vi "MainPannelFastEnabled - Copy.vi"() -> ()   [LabVIEW 2020]
uses:
  Digi/Controls/DigiMachineStates.ctl
  Digi/Digitizer_StatesMain.ctl
  <vilib>/userdefined/High Color/nirio_resource_hc.ctl
  Stage/New/StageOptions.ctl
  FileStore/Data Save State.ctl
  Gen/Generator_States.ctl
  <vilib>/Heliosphere Research LLC/Advanced Plotting Toolkit/properties/Colormap_Map.ctl
  <vilib>/Native 3D Graph/xcontrol/3DPC_SurfacePlot.xctl
  WaveClusterPacket.ctl
  <vilib>/UPVI/lvhdf5/library.llb/HDF5 Ref.ctl
  LongShotStates.ctl
  ImageCluster.ctl
  <vilib>/Platform/TimedLoop/XDataNode/timing_clust.ctl
  <vilib>/Platform/TimedLoop/XDataNode/nitl_modes.ctl
  <vilib>/Platform/TimedLoop/XDataNode/wakeup.ctl
  Stage/New/SettingCtrlOptions.ctl
  Stage/New/PosCtrlOptions.ctl
  Digi/Controls/FPGA VI Reference.ctl
  <extravilib>/ChannelInstances/Tag-bool/Read With Abort.vi
  <extravilib>/ChannelInstances/Tag-bool/Write.vi
  <extravilib>/ChannelInstances/Tag-bool/Write With Abort.vi
  <extravilib>/ChannelInstances/Tag-bool/Instantiate.vi
  <extravilib>/ChannelInstances/Tag-bool/EndpointRead.vi
  <vilib>/FPGAPlugInAG/PXIe-7962R/niLvFpga_Open_PXIe-7962R.vi
  <vilib>/rvi/interface/common/dynamic/niFpgaDynamicAddResources.vi
  <vilib>/FPGAPlugInAG/Dynamic/niLvFpga_Close_Dynamic.vi
  <extravilib>/ChannelInstances/Tag-bool/Endpoint.vi
  <vilib>/Platform/TimedLoop/XDataNode/XDataNode.xnode
  <vilib>/rvi/interface/nirviOpenFPGA/nirviOpenFPGA.xnode
  FPGA Bitfiles/DigitizerFPGACode(Fully_Functional)_v3.lvbitx
  <vilib>/rvi/interface/nirviCloseFPGA/nirviCloseFPGA.xnode
  <instrlib>/_niInstr/Basic Elements/v1/FPGA/niInstr Basic Elements v1 FPGA.lvlib
  <vilib>/Platform/TimedLoop/XDataNode/XDNodeRunTimeDep.lvlib
  Stage/libximc.lvlib
  <extravilib>/ChannelInstances/Tag-bool.lvlib
  <vilib>/Heliosphere Research LLC/Advanced Plotting Toolkit/Advanced Plotting Toolkit.lvlib
panel:
  in  "Save Img":bool
  out "Image Display":dbl[][](graph)
  in  "Colormap Selector":T1(ring)=enum."gray"
  in  "LongShot":bool
  out "Z Open?":bool
  out "Z Position":dbl format="%#.3g"
  in  "Z_Stop":bool
  in  "Z_MoveDown":bool
  in  "Z_Move Up":bool
  in  "Z_Step":dbl
  in  "Reset Button":bool
  in  "LogMode":bool
  in  "Start Digitizer UI Bttn":bool
  out "Max Index (s)":dbl format="%#_3p"
  out "Max Val (V)":dbl format="%#_3p"
  in  "Delay_Scroll_Range":dbl=2.0 caption="Range"
  in  "FineDelayControl":dbl(slide)=1.0 step=0.1 scale=-2.0..2.0
  in  "Amplitude Range":cluster{"Slider 1":dbl, "Slider 1":dbl}(slide)={"Slider 1"=1.0, "Slider 1"=1.6299559471365639} scale=-2.5..2.5
  in  "Pause Triggger":bool caption="Pause"
  in  "Delay(us)":sgl min=0 step=0.1 format="%#_4g"
  in  "Time Division":u8(slide)=1 max=2 step=1 scale=0.0..2.0
  in  "Amplitude \nAveraging":u16(slide)=1 caption="Amplitude Averaging" scale=0.0..7.0 scale format="%#.2g"
  in  "Record Size":u16=1024
  in  "RIO Resource":T2="PXI1Slot2"
  out "Configured?":bool
  out "TIS Configured?":bool
  out "Range (Vpp)":dbl=1.3
  out "Digitizer On":bool
  out "Waveform [LIVE]":cluster{"Start Time":dbl, dbl, ext[]}(graph)
  in  "TriggerDigi":bool
  in  "Scanning":bool
  in  "Single Shot":bool
  in  "LIVE":bool
  in  "Transducer Freq (Hz)":u64
  in  "Temperature (C)":dbl
  in  "Remarks":string
  in  "Immersion Medium":string
  in  "EXIT APP":bool
  in  "Save to File":bool=TRUE caption="Checkbox"
  out "No Trig Miss":bool
  in  "FileName":string
  in  "File Store Directory":path
  out "File Open?":bool
  out "X Step Size (R)":sgl format="%#_2g"
  out "Y Step Size (R)":sgl format="%#_2g"
  out "Scan Time (Approx.)":string
  out "Total Pixels":i32
  out "Moving?":bool
  out "Stage Position":cluster{sgl[], sgl[]}(graph) caption="XY Graph - Dark"
  in  "X Position Abs":dbl caption="X Position"
  in  "Y Position Abs":dbl caption="Y Position"
  out "Line Count":i32=6 caption="Y Pixels"
  out "Pixel Count":i32=6 caption="X Pixels"
  in  "X Start":sgl
  in  "X End":sgl=10.0
  in  "Y Start":sgl
  in  "Y End":sgl=8.0
  in  "Y Step Size":sgl=0.5
  in  "X Step Size":sgl=0.5
  in  "Scan Mode":enum16{"Raster", "Serpentine"}(ring)
  in  "Speed Control (mm/s)":sgl(slide)=4.0 min=0.1 scale=0.1..5.0
  in  "AbsMove":bool
  in  "Outline":bool
  in  "Start Stage":bool
  in  "Stop Motion":bool
  in  "Zero":bool
  in  "Right":bool
  in  "Left":bool
  in  "Move to Start":bool
  in  "Down":bool
  in  "Up":bool
  out "X Position":dbl format="%#.3g"
  out "Y Position":dbl format="%#.3g"
  in  "Move Step":dbl=1.0
  in  "Stop Stage":bool
  out "Controller Open?":bool
  in  "Developer Options Control":T3(tab)
  in  "Stop Gen App":bool
  out "Gen State":T4
  out "Error Out Gen":errorcluster
  in  "Send vi Trig":bool
  out "Gain":dbl
  out "Offset Factor":dbl
  out "Amplitudes":dbl[](array[numeric]) format="%.2f"
  out "Sampling Frequency (Hz)":u64
  out "Waves per Pixel":u32
  in  "Ext/nViTrig":bool=TRUE
  in  "Machine Mode":T5(ring)=enum."Normal"
  in  "Stop Stage App":bool
  out "Error Out Stage":errorcluster
  in  "Next Coordinate Index":i32
  in  "EdgePt/nPixelMap":bool=TRUE
  out "Coordinate Array":sgl[][](array[numeric])
  out "Step Sizes":sgl[](array[numeric])
  out "Peripheral Coordis":sgl[][](array[numeric])=[[0.0, 0.0], [1.8, 0.0], [3.6, 0.0], [5.3999996, 0.0], [7.2, 0.0], [9.0, 0.0], [9.0, 2.0], [7.2, 2.0], [5.3999996, 2.0], [3.6, 2.0], [1.8, 2.0], [0.0, 2.0], [0.0, 4.0], [1.8, 4.0], [3.6, 4.0], [5.3999996, 4.0], [7.2, 4.0], [9.0, 4.0], [9.0, 6.0], [7.2, 6.0], [5.3999996, 6.0], [3.6, 6.0], [1.8, 6.0], [0.0, 6.0], [0.0, 8.0], [1.8, 8.0], [3.6, 8.0], [5.3999996, 8.0], [7.2, 8.0], [9.0, 8.0], [9.0, 10.0], [7.2, 10.0], [5.3999996, 10.0], [3.6, 10.0], [1.8, 10.0], [0.0, 10.0]]
  in  "Correction Table Path (Hidden)":path
  out "Serial nos":u32[](array[numeric])
  out "Calibration":cluster{dbl, "MicrostepMode":u32}[](array[cluster])
  out "IDs":i32[](array[numeric])
  in  "X Max Stage":dbl=220.0 format="%#_13g"
  in  "Y Maximum":dbl=220.0
  out "Stage Status":T6
  out "Wave Count Zero":bool
  in  "CountReset":bool
  in  "Trigger Digi Single":bool
  in  "Start Digi":bool
  in  "Stop Digi App":bool caption="Stop Digi \nApplication"
  in  "Digi Machine Mode":T7=enum."Single Shot Mode"
  out "Waves Count":u32
  in  "Imaging":bool
  out "Digi State":T8
  out "nDigiLoopRunning":bool
  out "error out Digi":errorcluster
  out "Wave out packet":T9
  out "Error Out FileIO":errorcluster
  in  "Done Recording":bool
  in  "Record Data":bool
  in  "Open File":bool
  in  "Stop File App":bool
  out "FileStore State":T10
  out "Scan Running":bool=TRUE
  out "Scan Complete":bool=TRUE
  out "AmplitudeArray":dbl[](array[numeric])
  out "IndexArray":dbl[](array[numeric])
  in  "Map":T11
  in  "ColorBar":bool
  in  "Axis":bool
  out "Scanned Image":picture
  out "Topography Plot":refnum<class "Base Datatype.lvclass">[](xcontrol)
  in  "LongShotTimes":u8
  out "FilenameSimeStamped":string
  out "FileDirectoryFinal":path
  in  "Generator  Port":refnum<k15>
  out "Actual Sample Rate":dbl format="%#_6p"
  in  "Use Default Wave Settings":bool caption="Checkbox"
  in  "Start Gen":bool
  in  "stop Gen":bool
  out "Generator On":bool
  out "Input Waveform":dbl[](graph)
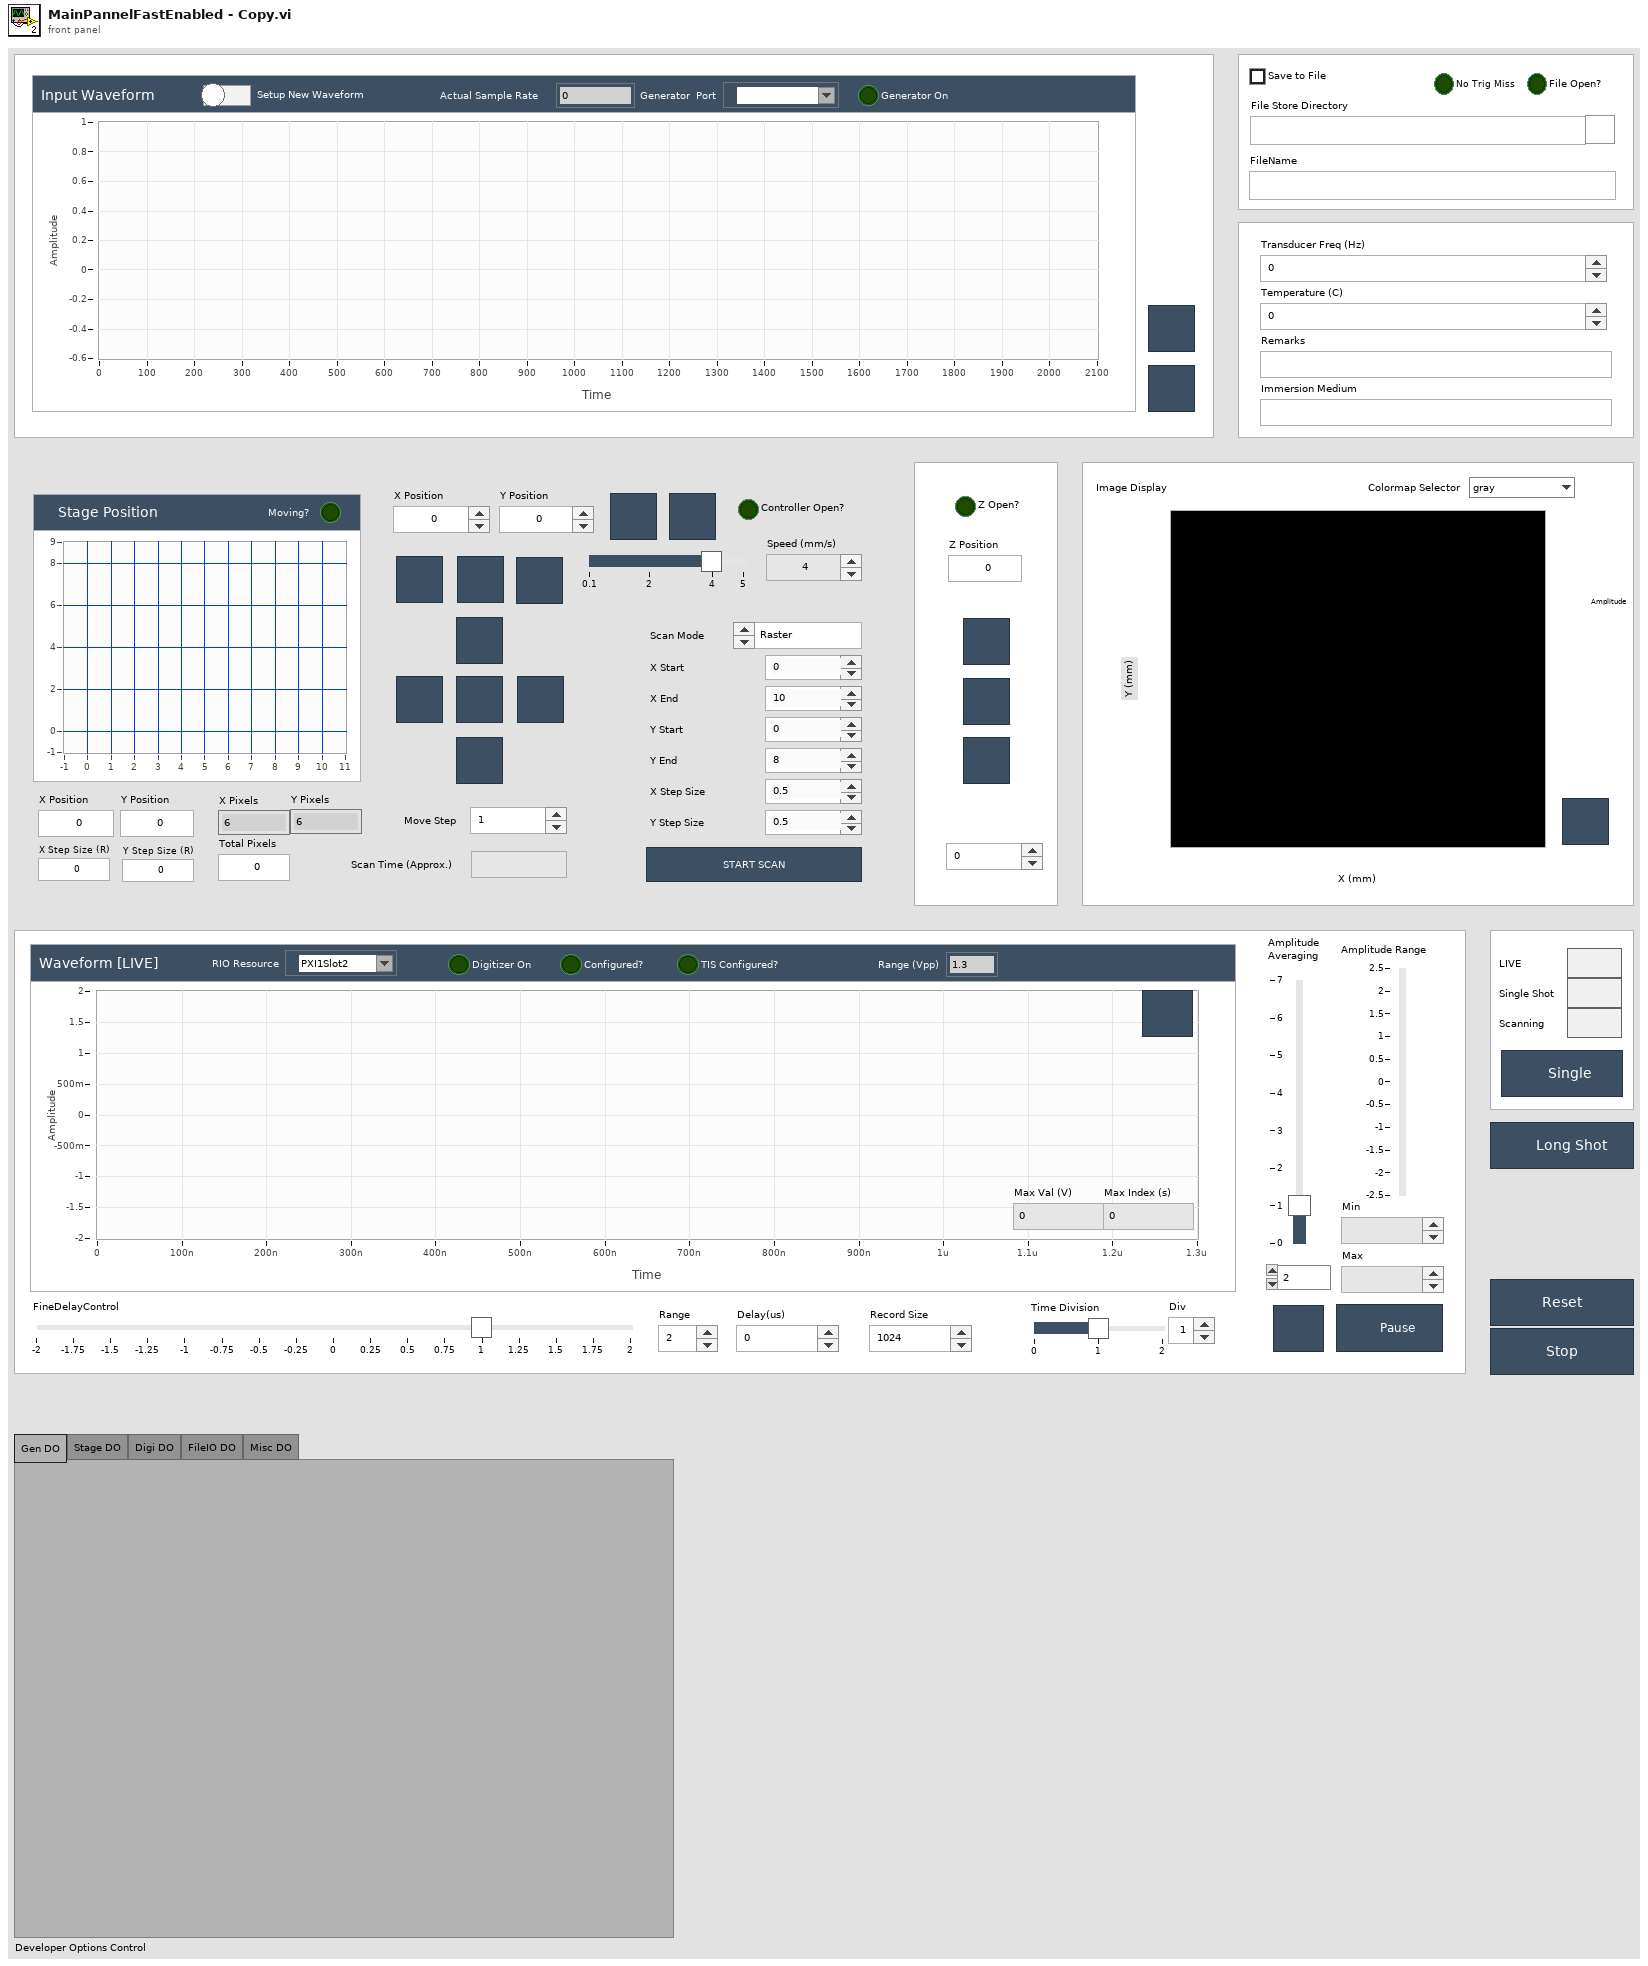
[diagram p1: front panel]
types:
  T1 = enum16{"fire", "rainbow", "gray", "inverse gray", "ice", "original"}
  T2 = typedef "nirio_resource_hc.ctl" = tag
  T3 = enum32{"Gen DO", "Stage DO", "Digi DO", "FileIO DO", "Misc DO"}
  T4 = typedef "Generator_States.ctl" = enum16{"Idle", "GenerateWaveArray", "InitGen", "SendVITrig", "CloseGen", "CloseApp"}
  T5 = enum16{"Scanning Mode", "Perimeter Mode", "Normal"}
  T6 = typedef "StageOptions.ctl" = enum16{"Idle", "Init", "Set Speed", "GenerateMotionPoints", "Scan_Start", "Scan_MoveNext", "Scan_SyncSet", "Scan_Get Pos", "Scan_Complete", "Cmd_MoveAbs", "Cmd_CloseControllers", "Cmd_MoveUp", "Cmd_MoveDown", "Cmd_MoveLeft", "Cmd_MoveRight", "Cmd_MoveStart", "Cmd_MoveZero", "Cmd_GetPos", "Cmd_Stop", "Sync_On", "Sync_Off", "Stop Motion", "CloseApplication"}
  T7 = typedef "DigiMachineStates.ctl" = enum16{"Scanning Mode", "Live Mode", "Single Shot Mode", "Idle Mode"}
  T8 = typedef "Digitizer_StatesMain.ctl" = enum16{"Idle", "Init", "SetParam", "VITrig", "Read", "CloseDigi", "CloseApp"}
  T9 = typedef "WaveClusterPacket.ctl" = cluster{"Wave Count":u32, "Wave":i16[]}
  T10 = typedef "Data Save State.ctl" = enum16{"Idle", "Open File", "Write Attributes", "Append Data", "Close File", "Close App"}
  T11 = typedef "Advanced Plotting Toolkit.lvlib/Colormap_Map.ctl" = enum16{"Automatic", "Rainbow", "Hot and Cold", "White-Black", "White-Blue", "White-Green", "White-Red", "Fire", "Water", "Earth", "Air", "Pastel", "Banded", "Stepped"}
  T12 = typedef "ImageCluster.ctl" = cluster{"Wave Count":i16, "Amplitude":i32, "Index":i32}
  T13 = typedef "LongShotStates.ctl" = enum16{"Idle", "Start Gen", "Set Digi Mode", "Clear Wave Count", "Set Initial Param", "Set Param", "Take Shot", "UpdateParam", "Show Data"}
  T14 = typedef "HDF5 Ref.ctl" = refnum<k1>
  T15 = typedef "XDNodeRunTimeDep.lvlib/timing_clust.ctl" = cluster{"Expected End [f-1]":u64, "Actual End [f-1]":u64, "Finished Late? [f-1]":bool, "Expected End [i-1]":u64, "Actual End [i-1]":u64, "Finished Late? [i-1]":bool, "Expected Start [i]":u64, "Actual Start [i]":u64, "Expected Start [f]":u64, "Actual Start [f]":u64, "Source Name":string, "Structure Name":string, "Period":i64, "Deadline":i64, "Offset":i64, "Start":i64, "Priority":i32, "Timeout":i32, "Mode":T16, "Wakeup Reason":T17, "Error":errorcluster, "Source Type":string, "Secondary Source Type":string, "Global End Time":u64, "Global Start Time":u64, "Frame Duration":u64, "Iteration Duration":u64, "Assigned CPU":i32, "I/O Scan Engine Mode":u32}
  T16 = typedef "XDNodeRunTimeDep.lvlib/nitl_modes.ctl" = enum32{"No Change", "Process missed periods, maintain original phase", "Discard missed periods, maintain original phase", "Process missed periods, ignore original phase", "Discard missed periods, ignore original phase"}
  T17 = typedef "XDNodeRunTimeDep.lvlib/wakeup.ctl" = enum32{"Normal", "Aborted", "Asynchronous wakeup", "Timing source error", "Timed loop error", "Timeout"}
  T18 = typedef "SettingCtrlOptions.ctl" = enum16{"Set X", "Set Y", "Set X and Y", "Get Settings", "None"}
  T19 = typedef "PosCtrlOptions.ctl" = enum16{"Move X", "Move Y", "Both X and Y", "Read Pos", "None"}
  T20 = typedef "imagedata.ctl" = cluster{"image type":i32, "image depth":i32, "image":u8[], "mask":u8[], "colors":u32[], "Rectangle":cluster{"left":i16, "top":i16, "right":i16, "bottom":i16}}
  T21 = typedef "FPGA VI Reference.ctl" = refnum<k20>
  T22 = typedef "Tag-bool.lvlib/))Channel.ctl" = refnum<queue>
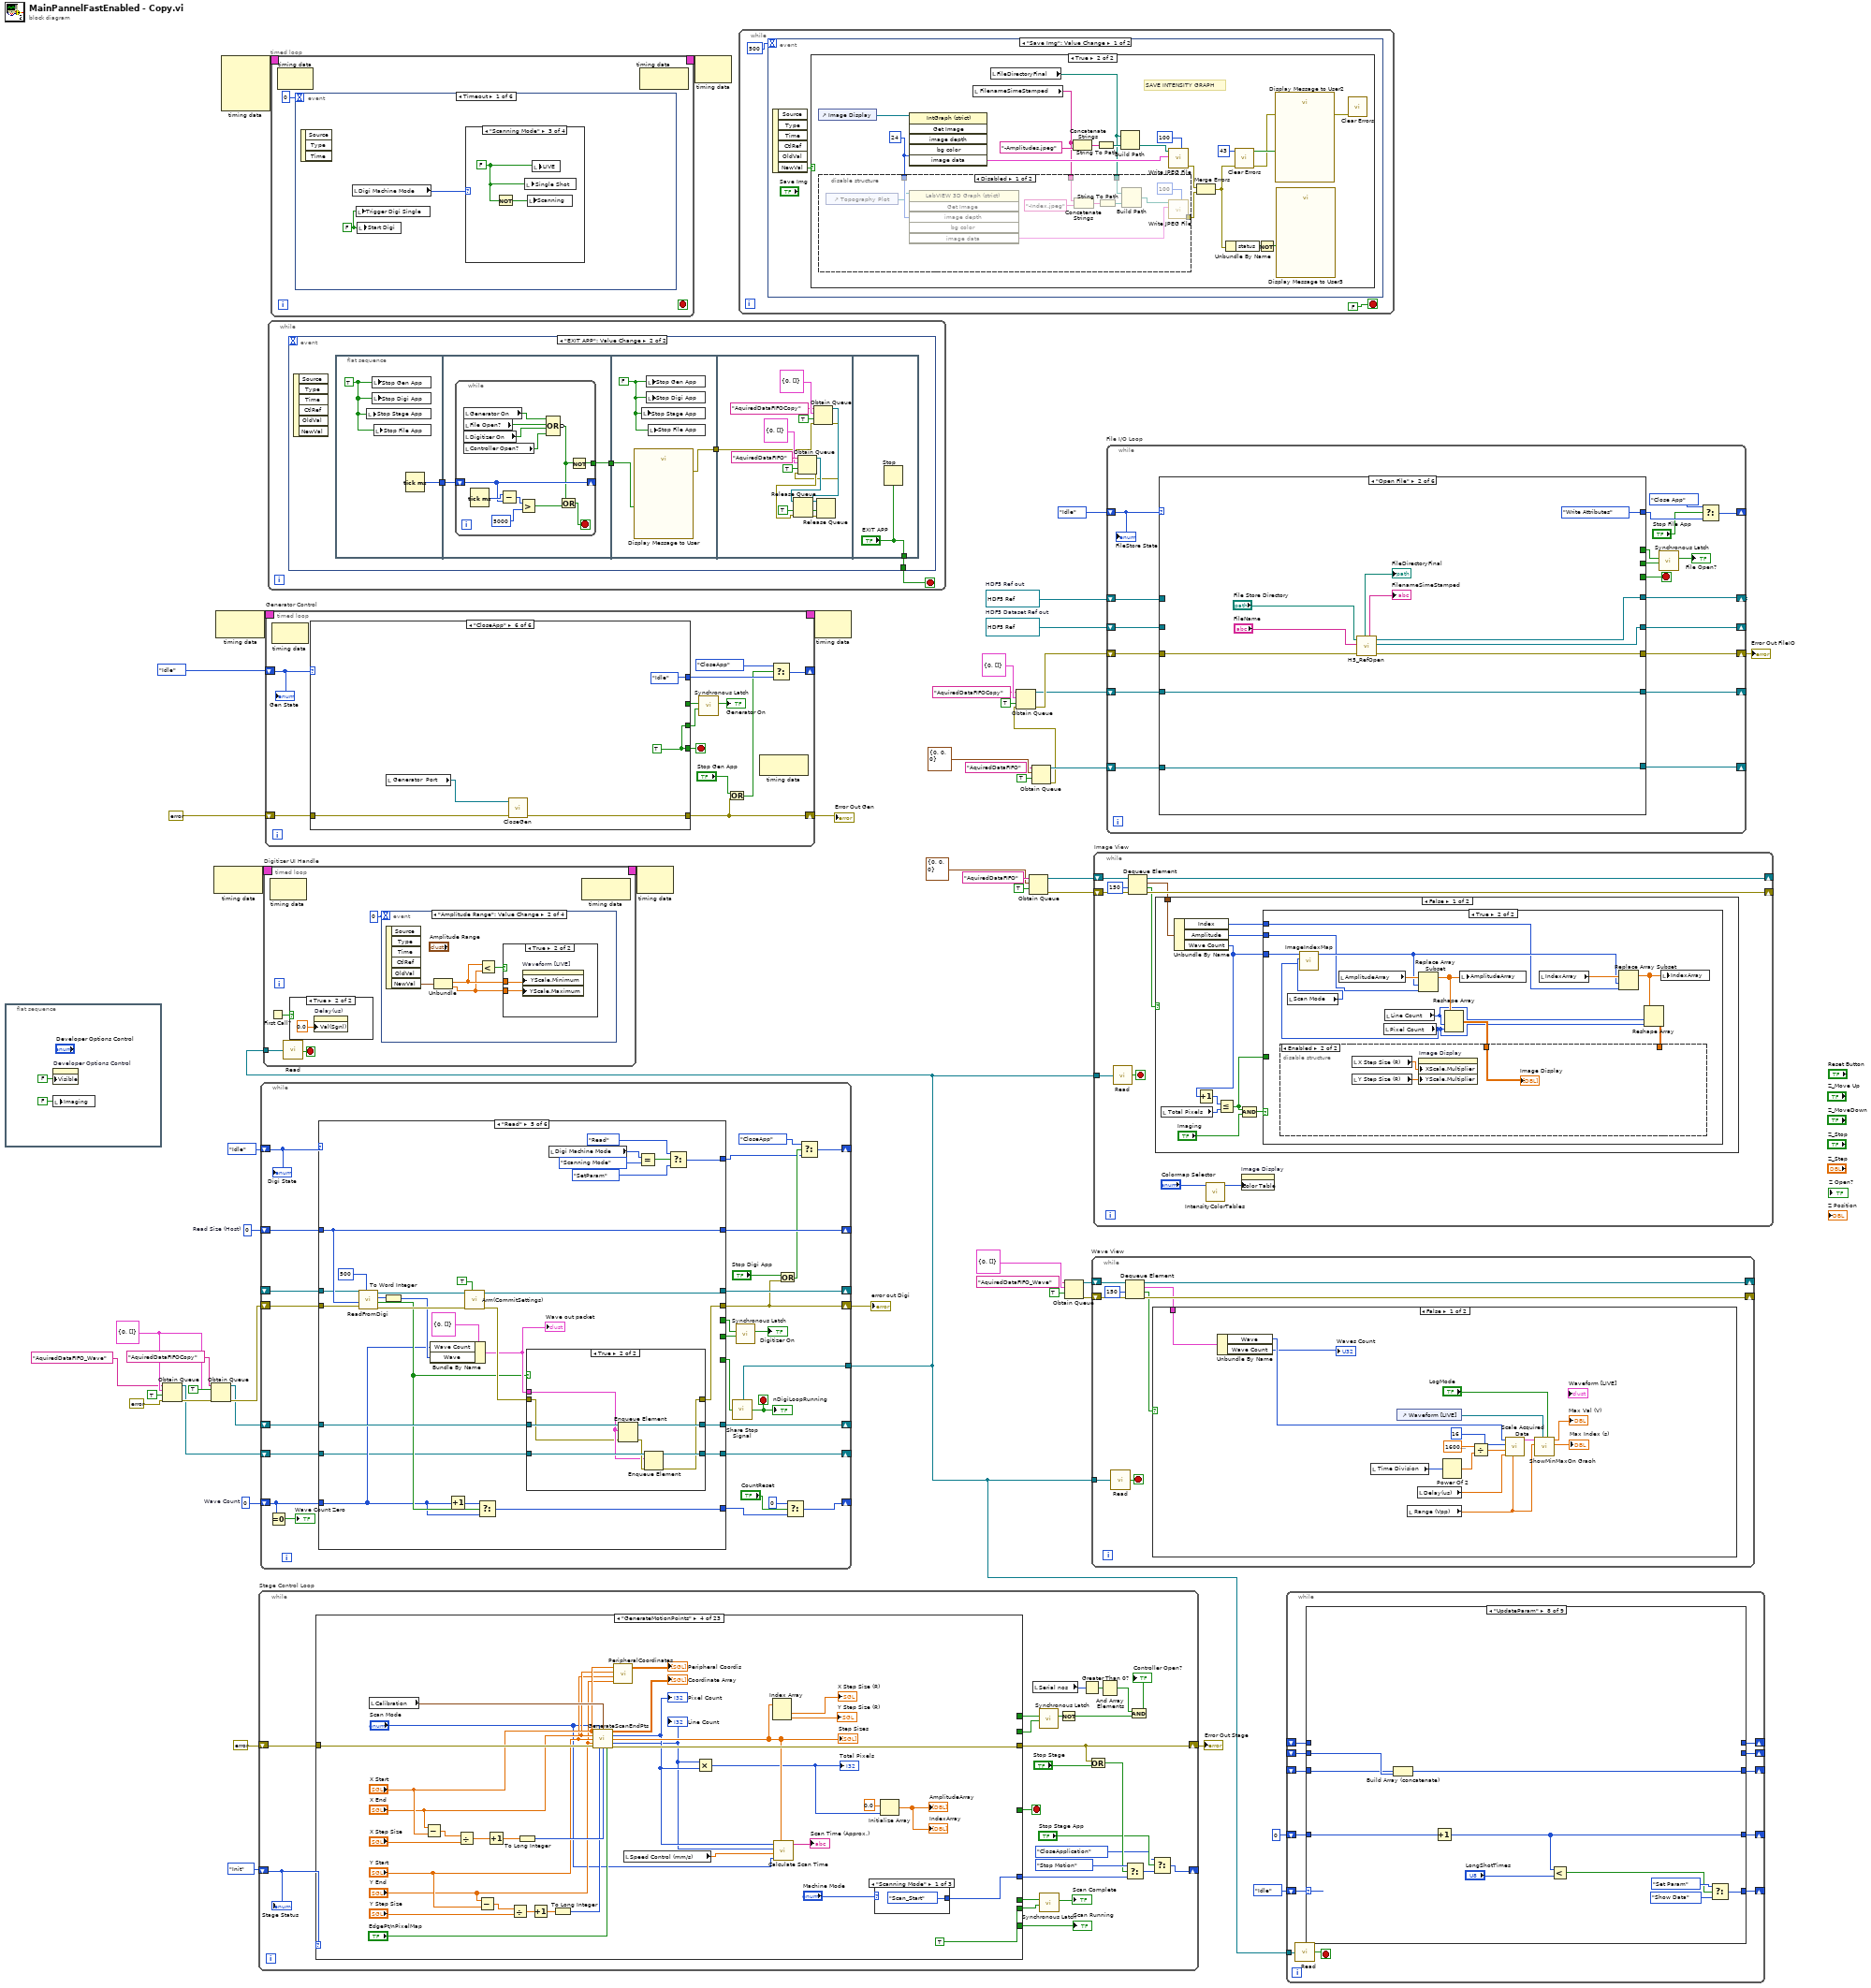
[diagram p0: block diagram]
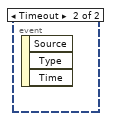
[diagram p4: hidden frame]
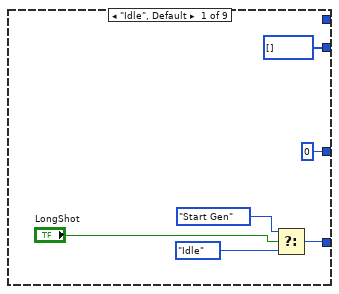
[diagram p5: hidden frame]
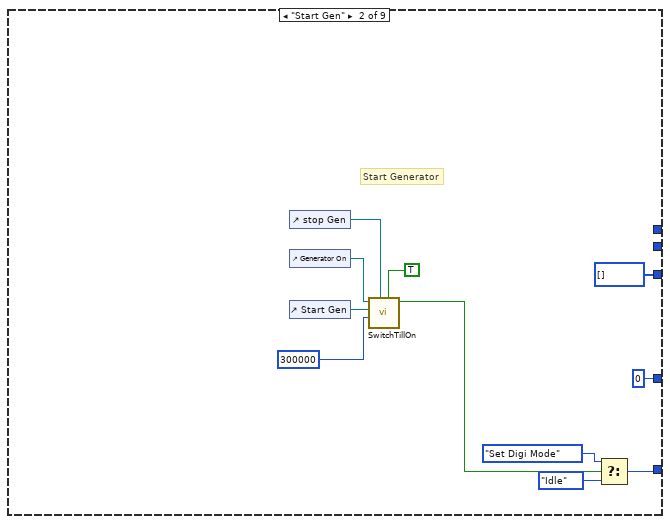
[diagram p6: hidden frame]
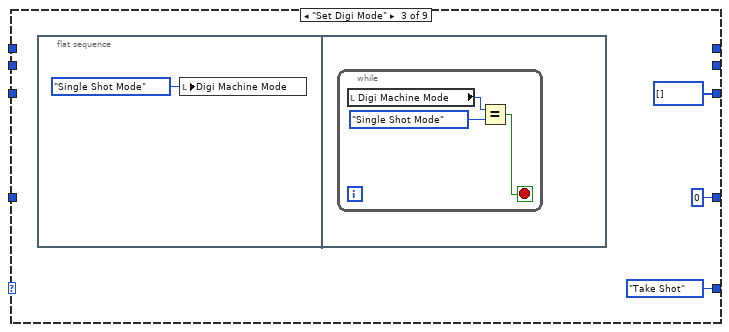
[diagram p7: hidden frame]
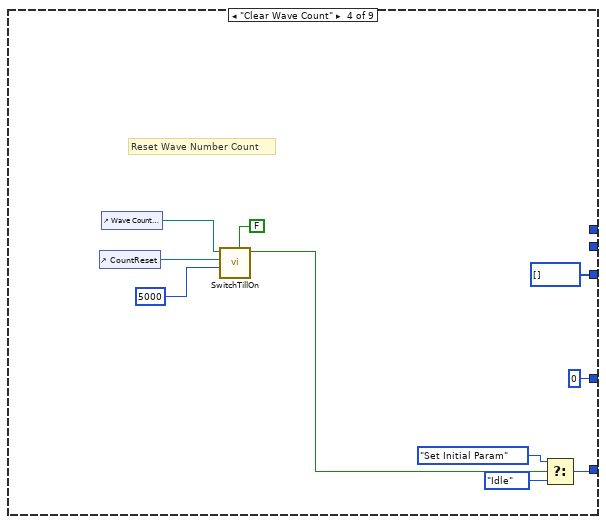
[diagram p8: hidden frame]
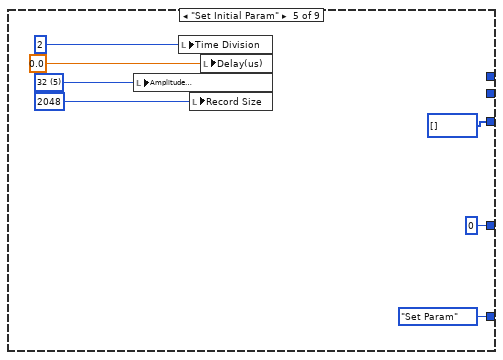
[diagram p9: hidden frame]
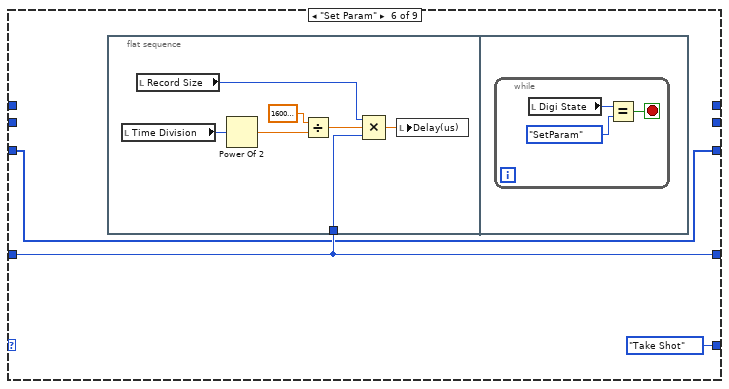
[diagram p10: hidden frame]
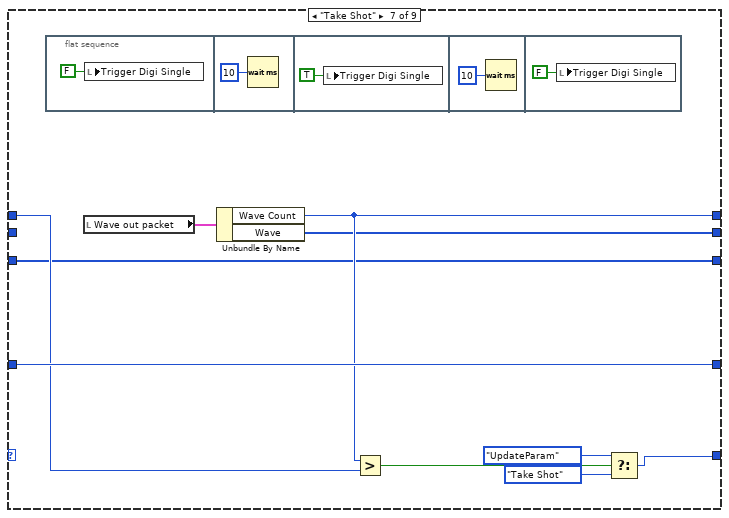
[diagram p11: hidden frame]
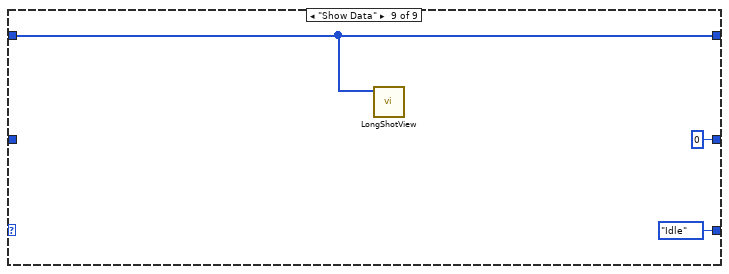
[diagram p12: hidden frame]
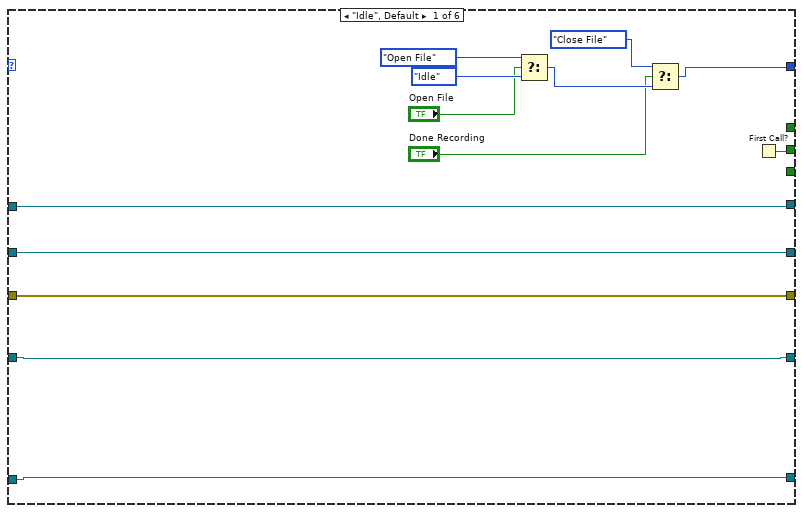
[diagram p14: hidden frame]
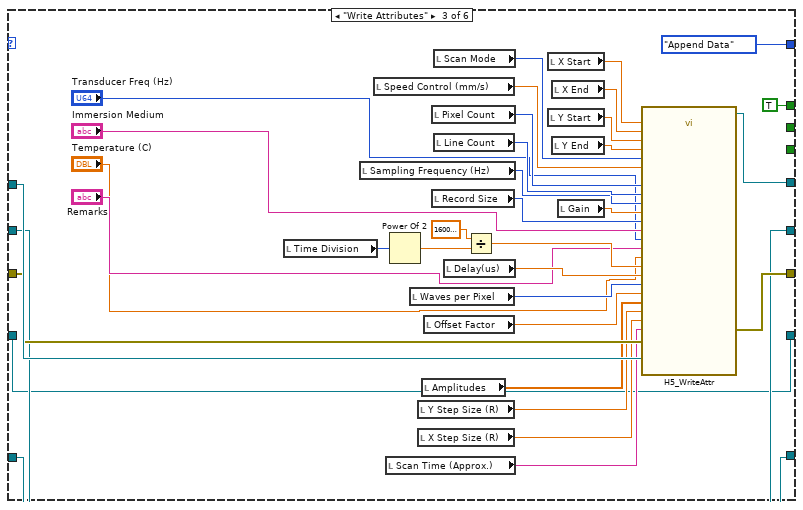
[diagram p15: hidden frame]
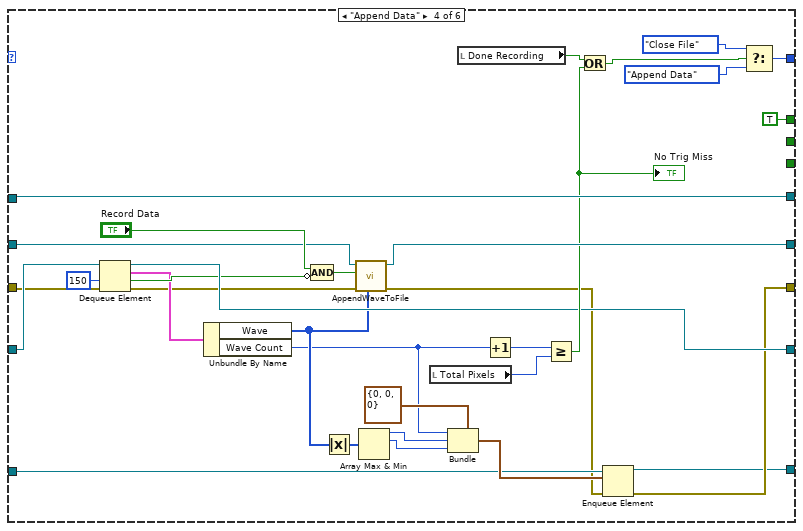
[diagram p16: hidden frame]
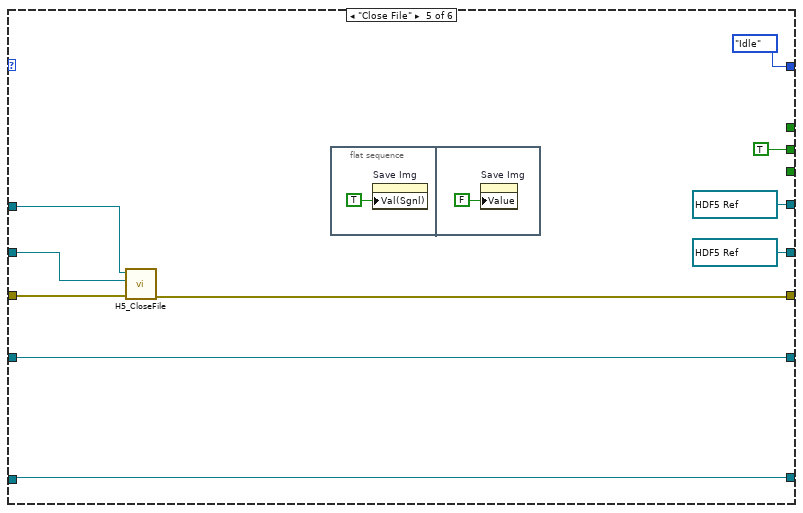
[diagram p17: hidden frame]
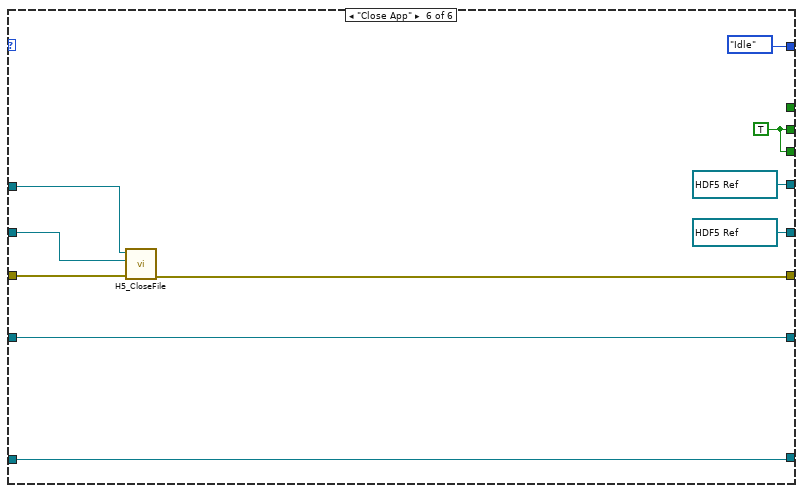
[diagram p18: hidden frame]
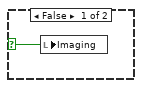
[diagram p19: hidden frame]
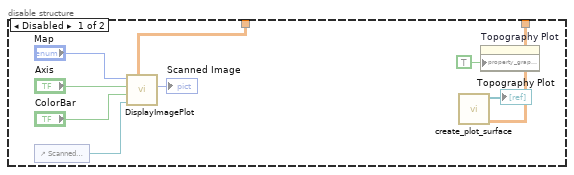
[diagram p20: hidden frame]
diagram:
  w31 = u16 0  # Wave Count
  w18 = T9 {"Wave Count"=0, "Wave"=[]} ("input cluster")
  w37 = T14 refnum items=["HDF5 Ref"]  # HDF5 Dataset Ref out
  w38 = T14 refnum items=["HDF5 Ref"]  # HDF5 Ref out
  w48 = u16 0  # Read Size (Host)
  n1 = flat-sequence {
    frame #0 {
      n2 = property on="Developer Options Control" class="TabCtl (strict)"("Visible"=FALSE) -> ()  [unwired: 2 in, 2 out]
      n3 = local write "Imaging"(FALSE ("Imaging")) -> ()
    }
  }
  n4 = Obtain Queue(name (unnamed)="AquiredDataFIFO_Wave", element data type=w18, create if not found? (T)=TRUE, error in (no error)=errorcluster {"status"=FALSE, "code"=0, "source"=""}) -> (queue out=w19:refnum<queue>, error out=w22:errorcluster)  [unwired: 1 in, 1 out]
  n5 = Obtain Queue(name (unnamed)="AquiredDataFIFOCopy", element data type=w18, create if not found? (T)=TRUE, error in (no error)=w22) -> (queue out=w33:refnum<queue>, error out=w34:errorcluster)  [unwired: 1 in, 1 out]
  n6 = node-c288() -> (w51:T15)  [unwired: 1 in]
  n7 = node-c288() -> (w45:T15)  [unwired: 1 in]
  n8 = node-c288() -> (w24:T15)  [unwired: 4 in]
  n9 = while "Stage Control Loop" {
    shift-right: [w68] -> _
    shift-left: StageOptions."Init" -> [w79]
    shift-right: [w76] -> w11
    shift-left: errorcluster {"status"=FALSE, "code"=0, "source"=""} ("error out") -> [w77]
    stop <- w69 stop-if-true
    n10 = case shown="\"GenerateMotionPoints\"" w79 {
      tunnel: [w84 w180 w203 w240 w245 w375 w390 w404 w444 w466 w475 w482 w493 w503 w513 w522 w530 w545 w551 w562 w571 w579 w590] -> w76
      tunnel: w77 -> [w84 w178 w204 w239 w247 w376 w391 w405 w442 w467 w476 w481 w494 w504 w514 w523 w531 w546 w550 w563 w572 w578 w589]
      tunnel: [w83 StageOptions."Set Speed" StageOptions."GenerateMotionPoints" w224 w248 w366 StageOptions."Scan_MoveNext" w401 StageOptions."Idle" StageOptions."Idle" StageOptions."Idle" StageOptions."Idle" StageOptions."Idle" StageOptions."Idle" StageOptions."Idle" StageOptions."Idle" StageOptions."Idle" StageOptions."Idle" StageOptions."Idle" StageOptions."Idle" StageOptions."Idle" StageOptions."Idle" StageOptions."Idle"] -> w74
      tunnel: [_ _ _ _ _ _ _ _ _ _ _ _ _ _ _ _ _ _ _ _ _ w575 w585] -> w72
      tunnel: [_ w181 _ _ _ _ _ _ _ _ _ _ _ _ _ _ _ _ _ _ _ _ _] -> w70
      tunnel: [_ _ _ _ _ _ _ _ _ _ _ _ _ _ _ _ _ _ _ _ _ _ w585] -> w69
      tunnel: [_ _ _ _ _ _ _ _ TRUE ("X SyncOut Enabled") _ _ _ _ _ _ _ _ _ _ _ _ _ _] -> w59
      tunnel: [TRUE ("EdgePt/nPixelMap") TRUE ("EdgePt/nPixelMap") TRUE ("EdgePt/nPixelMap") TRUE ("EdgePt/nPixelMap") TRUE ("EdgePt/nPixelMap") _ _ _ _ _ _ _ _ _ _ _ _ _ _ _ _ _ _] -> w57
      tunnel: [_ _ _ _ _ TRUE ("Moving?") TRUE ("Moving?") w392 FALSE ("Moving?") _ _ _ _ _ _ _ _ _ _ _ _ _ _] -> w56
      frame "Idle", Default {
        n11 = First Call?() -> (First Call?: T/F=w81:bool)
        n12 = event shown="[1] \"Up\": Value Change" {
          selector: _ -> [_ _ _ _ _ _ _ _ _ _ _ _ _]
          dyn-events: _ -> [_ _ _ _ _ _ _ _ _ _ _ _ _]
          timeout: 100 -> [_ _ _ _ _ _ _ _ _ _ _ _ _]
          tunnel: [w87 StageOptions."Cmd_MoveUp" StageOptions."Cmd_MoveDown" StageOptions."Cmd_MoveStart" StageOptions."Cmd_MoveLeft" StageOptions."Cmd_MoveRight" StageOptions."Cmd_MoveZero" StageOptions."Cmd_Stop" StageOptions."GenerateMotionPoints" StageOptions."GenerateMotionPoints" StageOptions."Set Speed" w159 StageOptions."Cmd_MoveAbs"] -> w83
          event Timeout {
            n13 = event-data() -> ()  [unwired: 1 in, 3 out]
            n14 = local read "Controller Open?"() -> (w88:bool)
            n15 = case shown="False" w88 {
              tunnel: [StageOptions."Init" StageOptions."Cmd_GetPos"] -> w87
              frame False {
              }
              frame True {
              }
            }
          }
          event "Up": Value Change {
            w91 = 0.0  # Y Start
            w93 = sgl 0.0  # X Start
            w96 = 1.0  # Offset
            n16 = event-data() -> ()  [unwired: 1 in, 6 out]
            n17 = local read "X Max Stage"() -> (w94:dbl)
            n18 = local read "Y Maximum"() -> (w92:dbl)
            n19 = Add(x=w96, y=w94) -> (x+y=w98:dbl)
            n20 = Subtract(x=w93, y=w96) -> (x-y=w99:dbl)
            n21 = Subtract(x=w91, y=w96) -> (x-y=w95:dbl)
            n22 = Add(x=w92, y=w96) -> (x+y=w97:dbl)
            n23 = Build Array(w93, w94) -> (w101:dbl[])
            n24 = Build Array(w91, w92) -> (w100:dbl[])
            n25 = property on="Stage Position" class="XYGraph (strict)"("XScale.Maximum"=w98, "XScale.Minimum"=w99, "YScale.Maximum"=w97, "YScale.Minimum"=w95, "XScale.MarkerVals[]"=w101, "YScale.MarkerVals[]"=w100) -> ()  [unwired: 2 in, 2 out]
          }
          event "Down": Value Change {
            w103 = 0.0  # Y Start
            w105 = sgl 0.0  # X Start
            w108 = 1.0  # Offset
            n26 = event-data() -> ()  [unwired: 1 in, 6 out]
            n27 = local read "X Max Stage"() -> (w106:dbl)
            n28 = local read "Y Maximum"() -> (w104:dbl)
            n29 = Add(x=w108, y=w106) -> (x+y=w110:dbl)
            n30 = Subtract(x=w105, y=w108) -> (x-y=w111:dbl)
            n31 = Subtract(x=w103, y=w108) -> (x-y=w107:dbl)
            n32 = Add(x=w104, y=w108) -> (x+y=w109:dbl)
            n33 = Build Array(w105, w106) -> (w113:dbl[])
            n34 = Build Array(w103, w104) -> (w112:dbl[])
            n35 = property on="Stage Position" class="XYGraph (strict)"("XScale.Maximum"=w110, "XScale.Minimum"=w111, "YScale.Maximum"=w109, "YScale.Minimum"=w107, "XScale.MarkerVals[]"=w113, "YScale.MarkerVals[]"=w112) -> ()  [unwired: 2 in, 2 out]
          }
          event "Move to Start": Value Change {
            n36 = event-data() -> ()  [unwired: 1 in, 6 out]
          }
          event "Left": Value Change {
            w116 = 0.0  # Y Start
            w118 = sgl 0.0  # X Start
            w121 = 1.0  # Offset
            n37 = event-data() -> ()  [unwired: 1 in, 6 out]
            n38 = local read "X Max Stage"() -> (w119:dbl)
            n39 = local read "Y Maximum"() -> (w117:dbl)
            n40 = Add(x=w121, y=w119) -> (x+y=w123:dbl)
            n41 = Subtract(x=w118, y=w121) -> (x-y=w124:dbl)
            n42 = Subtract(x=w116, y=w121) -> (x-y=w120:dbl)
            n43 = Add(x=w117, y=w121) -> (x+y=w122:dbl)
            n44 = Build Array(w118, w119) -> (w126:dbl[])
            n45 = Build Array(w116, w117) -> (w125:dbl[])
            n46 = property on="Stage Position" class="XYGraph (strict)"("XScale.Maximum"=w123, "XScale.Minimum"=w124, "YScale.Maximum"=w122, "YScale.Minimum"=w120, "XScale.MarkerVals[]"=w126, "YScale.MarkerVals[]"=w125) -> ()  [unwired: 2 in, 2 out]
          }
          event "Right": Value Change {
            w128 = 0.0  # Y Start
            w130 = sgl 0.0  # X Start
            w133 = 1.0  # Offset
            n47 = event-data() -> ()  [unwired: 1 in, 6 out]
            n48 = local read "X Max Stage"() -> (w131:dbl)
            n49 = local read "Y Maximum"() -> (w129:dbl)
            n50 = Add(x=w133, y=w131) -> (x+y=w135:dbl)
            n51 = Subtract(x=w130, y=w133) -> (x-y=w136:dbl)
            n52 = Subtract(x=w128, y=w133) -> (x-y=w132:dbl)
            n53 = Add(x=w129, y=w133) -> (x+y=w134:dbl)
            n54 = Build Array(w130, w131) -> (w138:dbl[])
            n55 = Build Array(w128, w129) -> (w137:dbl[])
            n56 = property on="Stage Position" class="XYGraph (strict)"("XScale.Maximum"=w135, "XScale.Minimum"=w136, "YScale.Maximum"=w134, "YScale.Minimum"=w132, "XScale.MarkerVals[]"=w138, "YScale.MarkerVals[]"=w137) -> ()  [unwired: 2 in, 2 out]
          }
          event "Zero": Value Change {
            w140 = 0.0  # Y Start
            w142 = sgl 0.0  # X Start
            w145 = 1.0  # Offset
            n57 = event-data() -> ()  [unwired: 1 in, 6 out]
            n58 = local read "X Max Stage"() -> (w143:dbl)
            n59 = local read "Y Maximum"() -> (w141:dbl)
            n60 = Add(x=w145, y=w143) -> (x+y=w147:dbl)
            n61 = Subtract(x=w142, y=w145) -> (x-y=w148:dbl)
            n62 = Subtract(x=w140, y=w145) -> (x-y=w144:dbl)
            n63 = Add(x=w141, y=w145) -> (x+y=w146:dbl)
            n64 = Build Array(w142, w143) -> (w150:dbl[])
            n65 = Build Array(w140, w141) -> (w149:dbl[])
            n66 = property on="Stage Position" class="XYGraph (strict)"("XScale.Maximum"=w147, "XScale.Minimum"=w148, "YScale.Maximum"=w146, "YScale.Minimum"=w144, "XScale.MarkerVals[]"=w150, "YScale.MarkerVals[]"=w149) -> ()  [unwired: 2 in, 2 out]
          }
          event "Stop Motion": Value Change {
            n67 = event-data() -> ()  [unwired: 1 in, 6 out]
          }
          event "Start Stage": Value Change {
            n68 = event-data() -> ()  [unwired: 1 in, 6 out]
            n69 = local write "Machine Mode"(T5."Scanning Mode" ("Machine Mode")) -> ()
          }
          event "X Start", "X End", "Y Start", "Y End", "Y Step Size", "X Step Size", "Scan Mode": Value Change {
            n70 = event-data() -> ()  [unwired: 1 in, 6 out]
            n71 = local write "Machine Mode"(T5."Normal" ("Machine Mode")) -> ()
          }
          event "Speed Control (mm/s)": Value Change {
            n72 = event-data() -> ()  [unwired: 1 in, 6 out]
          }
          event "Outline": Value Change {
            n73 = event-data() -> ()  [unwired: 1 in, 6 out]
            n74 = case shown="True" "Outline" {
              tunnel: [StageOptions."Idle" StageOptions."GenerateMotionPoints"] -> w159
              frame False {
              }
              frame True {
                n75 = local write "Machine Mode"(T5."Perimeter Mode" ("Machine Mode")) -> ()
              }
            }
          }
          event "AbsMove": Value Change {
            w163 = 0.0  # Y Start
            w165 = sgl 0.0  # X Start
            w168 = 1.0  # Offset
            n76 = event-data() -> ()  [unwired: 1 in, 6 out]
            n77 = local read "X Max Stage"() -> (w166:dbl)
            n78 = local read "Y Maximum"() -> (w164:dbl)
            n79 = Add(x=w168, y=w166) -> (x+y=w170:dbl)
            n80 = Subtract(x=w165, y=w168) -> (x-y=w171:dbl)
            n81 = Subtract(x=w163, y=w168) -> (x-y=w167:dbl)
            n82 = Add(x=w164, y=w168) -> (x+y=w169:dbl)
            n83 = Build Array(w165, w166) -> (w173:dbl[])
            n84 = Build Array(w163, w164) -> (w172:dbl[])
            n85 = property on="Stage Position" class="XYGraph (strict)"("XScale.Maximum"=w170, "XScale.Minimum"=w171, "YScale.Maximum"=w169, "YScale.Minimum"=w167, "XScale.MarkerVals[]"=w173, "YScale.MarkerVals[]"=w172) -> ()  [unwired: 2 in, 2 out]
          }
        }
        n86 = case shown="True" w81 {
          frame False {
          }
          frame True {
            # "Trigger the Time Output\nFor the default values"
            n87 = property on="Scan Mode" class="Enum (strict)"() -> ("Value"=w86:enum16{"Raster", "Serpentine"})  [unwired: 2 in, 2 out]
            n88 = property on="Scan Mode" class="Enum (strict)"("Val(Sgnl)"=w86) -> ()  [unwired: 2 in, 2 out]
            n89 = local write "Machine Mode"(T5."Normal" ("Machine Mode")) -> ()
          }
        }
      }
      frame "Init" {
        w187 = 100  # numSteps = 1mm
        w188 = TRUE  # Correction File Path Option
        n90 = call "CloseDevices.vi"("error in (no error)"=w178, "Close"=TRUE, "Ids"=i32[] [1, 2]) -> ("error out"=w177:errorcluster)  [unwired: 8 in]
        n91 = case shown="False" w188 {
          tunnel: ["Correction Table Path (Hidden)" w194] -> w189
          frame False {
          }
          frame True {
            w195 = path "Corr_table_8MT173-25.tbl"  # File Name
            n92 = Current VI's Path() -> (path=w197:path)
            n93 = Build Path(base path=w197, name or relative path=path "") -> (appended path=w196:path)
            n94 = Build Path(base path=w196, name or relative path=w195) -> (appended path=w194:path)
          }
        }
        n95 = call "Find Controllers.vi"("error in (no error)"=w177) -> ("error out"=w191:errorcluster, "Names"=w192:string[])  [unwired: 8 in, 1 out]
        n96 = call "OpenDevices.vi"("error In"=w191, "Names"=w192) -> ("error out"=w190:errorcluster, "Serial nos"=→"Serial nos":u32[], "IDs"=w185:i32[])  [unwired: 6 in]
        "IDs" <- w185
        n97 = call "CalibrateStage.vi"("error in (no error)"=w190, "numSteps = 1mm"=w187, "Correction Table Path"=w189, "IDs"=w185) -> ("error out"=w180:errorcluster, "Calibration"=→"Calibration":cluster{dbl, "MicrostepMode":u32}[])  [unwired: 2 in, 4 out]
        n98 = Unbundle By Name(w180) -> ("status"=w182:bool)
        n99 = Not(x=w182) -> (.not. x?=w181:bool)
      }
      frame "Set Speed" {
        n100 = local read "IDs"() -> (w202:i32[])
        n101 = local read "Calibration"() -> (w201:cluster{dbl, "MicrostepMode":u32}[])
        n102 = call "SetMoveSettings.vi"("Mode"=SettingCtrlOptions."Set X and Y", "error in (no error)"=w204, "Calibration"=w201, "Speed"="Speed Control (mm/s)", "IDs"=w202) -> ("error out"=w203:errorcluster)  [unwired: 4 in, 2 out]
      }
      frame "GenerateMotionPoints" {
        n103 = local read "Calibration"() -> (w230:cluster{dbl, "MicrostepMode":u32}[])
        n104 = Subtract(x="X End", y="X Start") -> (x-y=w219:sgl)
        n105 = Divide(x=w219, y="X Step Size") -> (x/y=w235:sgl)
        n106 = Subtract(x="Y End", y="Y Start") -> (x-y=w217:sgl)
        n107 = Increment(x=w235) -> (x+1=w222:sgl)
        n108 = Divide(x=w217, y="Y Step Size") -> (x/y=w232:sgl)
        n109 = To Long Integer(number=w222) -> (32bit integer=w234:i32)
        n110 = Increment(x=w232) -> (x+1=w221:sgl)
        n111 = To Long Integer(number=w221) -> (32bit integer=w231:i32)
        n112 = call "GenerateScanEndPts.vi"("X Start"="X Start", "Mode"="Scan Mode", "Calibration In"=w230, "X End"="X End", "Y Start"="Y Start", "Y End"="Y End", "error in"=w239, "Line Count"=w231, "Pixel Count"=w234, "EdgePt/nPixelMap"="EdgePt/nPixelMap") -> ("Coordinate Array"=→"Coordinate Array":sgl[][], "X Pixel Count"=w213:i32, "Step Sizes"=w215:sgl[], "Y Pixel Count"=w212:i32, "error out"=w240:errorcluster)  [unwired: 1 in]
        "Line Count" <- w212
        "Pixel Count" <- w213
        "Step Sizes" <- w215
        n113 = call "PeripheralCoordinates.vi"("Y End"="Y End", "Y Start"="Y Start", "X End"="X End", "X Start"="X Start") -> ("Coordinate Array"=→"Peripheral Coordis":sgl[][])  [unwired: 7 in]
        n114 = local read "Speed Control (mm/s)"() -> (w216:sgl)
        n115 = Multiply(x=w212, y=w213) -> (x*y=w209:i32)
        "Total Pixels" <- w209
        n116 = Index Array(array=w215) -> (element #1=→"X Step Size (R)":sgl, element #2=→"Y Step Size (R)":sgl)  [unwired: 2 in]
        n117 = call "Calculate Scan Time.vi"("Step Sizes"=w215, "Scan Mode"="Scan Mode", "Speed Control (mm/s)"=w216, "Line Count"=w212, "Pixel Count"=w213) -> ("TimeString"=→"Scan Time (Approx.)":string)  [unwired: 2 in, 4 out]
        n118 = case shown="\"Scanning Mode\"" "Machine Mode" {
          tunnel: [StageOptions."Scan_Start" StageOptions."Scan_Start" StageOptions."Idle"] -> w224
          frame "Scanning Mode" {
          }
          frame "Perimeter Mode" {
          }
          frame "Normal", Default {
          }
        }
        n119 = Initialize Array(0.0 ("element"), w209) -> (→"AmplitudeArray" →"IndexArray":dbl[])
      }
      frame "Scan_Start" {
        n120 = call <vilib>:"Set Busy.vi"("error in (no error)"=w247) -> ("error out"=w246:errorcluster)  [unwired: 9 in, 1 out]
        n121 = stacked-sequence {
          seq-local: [_ w256 _ _ _ _ _] -> [_ _ _ _ _ _ w328]
          seq-local: [w250 _ _ _ _ _ _] -> [_ _ _ _ _ _ w329]
          seq-local: [_ _ _ _ w310 _ _] -> [_ _ _ _ _ _ w326]
          seq-local: [_ _ _ w282 _ _ _] -> [_ _ _ _ _ _ w327]
          seq-local: [_ _ _ _ _ w319 _] -> [_ _ _ _ _ _ w325]
          tunnel: w246 -> [_ _ _ _ _ _ w348]
          tunnel: [_ _ _ _ _ _ w342] -> w249
          tunnel: [_ _ _ _ _ _ w331] -> w248
          frame #0 {
            # "Start Generator"
            n122 = control-ref of="stop Gen"() -> (w252:refnum<vi>)
            n123 = control-ref of="Generator On"() -> (w254:refnum<vi>)
            n124 = control-ref of="Start Gen"() -> (w253:refnum<vi>)
            n125 = call "SwitchTillOn.vi"("Stop if On?"=TRUE, "Turn Off Button"=w252, "timeout"=u32 300000, "Turn On Button"=w253, "Turn On Indicator"=w254) -> ("Success?"=w250:bool)  [unwired: 6 in]
          }
          frame #1 {
            # "Start Digitizer"
            n126 = flat-sequence {
              tunnel: [w258] -> w257
              tunnel: w257 -> [w264]
              tunnel: [w264] -> w256
              frame #0 {
                n127 = control-ref of="Digitizer On"() -> (w261:refnum<vi>)
                n128 = control-ref of="Start Digi"() -> (w260:refnum<vi>)
                n129 = call "SwitchTillOn.vi"("Stop if On?"=FALSE, "timeout"=u32 5000, "Turn On Button"=w260, "Turn On Indicator"=w261) -> ("Success?"=w258:bool)  [unwired: 7 in]
              }
              frame #1 {
                n130 = local write "Digi Machine Mode"(DigiMachineStates."Scanning Mode" ("Digi Machine Mode")) -> ()
              }
              frame #2 {
                n131 = while {
                  stop <- w266 stop-if-true
                  n132 = local read "Digi Machine Mode"() -> (w267:T7)
                  n133 = Equal?(x=w267, y=DigiMachineStates."Scanning Mode") -> (x = y?=w266:bool)
                }
              }
            }
          }
          frame #2 {
            # "Reset Data Storing"
            n134 = flat-sequence {
              frame #0 {
                n135 = while {
                  stop <- w269 stop-if-true
                  n136 = local read "FileStore State"() -> (w273:T10)
                  n137 = local read "FileStore State"() -> (w271:T10)
                  n138 = local write "Done Recording"(TRUE ("Done Recording")) -> ()
                  n139 = Equal?(x=w271, y=Data_Save_State."Close File" ("FileStore State")) -> (x = y?=w268:bool)
                  n140 = Equal?(x=w273, y=Data_Save_State."Idle" ("FileStore State")) -> (x = y?=w272:bool)
                  n141 = Or(x=w272, y=w268) -> (x .or. y?=w269:bool)
                }
              }
              frame #1 {
                n142 = local write "Done Recording"(FALSE ("Done Recording")) -> ()
              }
            }
          }
          frame #3 {
            w278 = T9 {"Wave Count"=0, "Wave"=[]} ("input cluster")
            # "Flush All Queue"
            n143 = Obtain Queue(name (unnamed)="AquiredDataFIFO_Wave", element data type=w278, create if not found? (T)=TRUE) -> (queue out=w279:refnum<queue>, error out=w280:errorcluster)  [unwired: 2 in, 1 out]
            n144 = Obtain Queue(name (unnamed)="AquiredDataFIFOCopy", element data type=w278, create if not found? (T)=TRUE, error in (no error)=w280) -> (queue out=w287:refnum<queue>, error out=w285:errorcluster)  [unwired: 1 in, 1 out]
            n145 = Obtain Queue(name (unnamed)="AquiredDataFIFO", element data type=w278, create if not found? (T)=TRUE, error in (no error)=w285) -> (queue out=w288:refnum<queue>, error out=w286:errorcluster)  [unwired: 1 in, 1 out]
            n146 = while {
              tunnel: w288 -> [w309]
              tunnel: w287 -> [w308]
              shift-right: [w296] -> w284
              shift-left: w286 -> [w305]
              tunnel: w279 -> [w293]
              stop <- w298 stop-if-true
              n147 = Flush Queue(queue=w309, error in (no error)=w305) -> (queue out=w304:refnum<queue>, error out=w306:errorcluster)  [unwired: 1 out]
              n148 = Get Queue Status(queue=w304) -> (# elements in queue=w300:i32)  [unwired: 2 in, 7 out]
              n149 = Flush Queue(queue=w308, error in (no error)=w306) -> (queue out=w302:refnum<queue>, error out=w307:errorcluster)  [unwired: 1 out]
              n150 = Get Queue Status(queue=w302, error in (no error)=w307) -> (error out=w303:errorcluster, # elements in queue=w301:i32)  [unwired: 1 in, 6 out]
              n151 = Flush Queue(queue=w293, error in (no error)=w303) -> (queue out=w295:refnum<queue>, error out=w297:errorcluster)  [unwired: 1 out]
              n152 = Get Queue Status(queue=w295, error in (no error)=w297) -> (error out=w296:errorcluster, # elements in queue=w294:i32)  [unwired: 1 in, 6 out]
              n153 = Compound Arithmetic op=ADD(w294, w301, w300) -> (w299:i32)
              n154 = Equal To 0?(x=w299) -> (x = 0?=w298:bool)
            }
            n155 = Unbundle By Name(w284) -> ("status"=w283:bool)
            n156 = Not(x=w283) -> (.not. x?=w282:bool)
          }
          frame #4 {
            # "Open File"
            n157 = case shown="False" "Save to File" {
              tunnel: [TRUE ("Success?") w315] -> w310
              frame False {
              }
              frame True {
                n158 = control-ref of="Done Recording"() -> (w313:refnum<vi>)
                n159 = control-ref of="File Open?"() -> (w316:refnum<vi>)
                n160 = control-ref of="Open File"() -> (w317:refnum<vi>)
                n161 = call "SwitchTillOn.vi"("Stop if On?"=TRUE, "Turn Off Button"=w313, "timeout"=u32 5000, "Turn On Button"=w317, "Turn On Indicator"=w316) -> ("Success?"=w315:bool)  [unwired: 6 in]
                n162 = local write "Record Data"(w315) -> ()
              }
            }
          }
          frame #5 {
            # "Reset Wave Number Count"
            n163 = control-ref of="CountReset"() -> (w320:refnum<vi>)
            n164 = control-ref of="Wave Count Zero"() -> (w321:refnum<vi>)
            n165 = call "SwitchTillOn.vi"("Stop if On?"=FALSE, "timeout"=u32 5000, "Turn On Button"=w320, "Turn On Indicator"=w321) -> ("Success?"=w319:bool)  [unwired: 7 in]
          }
          frame #6 {
            w345 = 0.0 ("element")
            w354 = 1.0  # Offset
            # "Draw Markers To Indicate the Scan Area"
            n166 = property on="X End" class="DigNum (strict)"() -> ("Value"=w353:sgl)  [unwired: 2 in, 2 out]
            n167 = property on="X Start" class="DigNum (strict)"() -> ("Value"=w352:sgl)  [unwired: 2 in, 2 out]
            n168 = property on="Y End" class="DigNum (strict)"() -> ("Value"=w349:sgl)  [unwired: 2 in, 2 out]
            n169 = property on="Y Start" class="DigNum (strict)"() -> ("Value"=w351:sgl)  [unwired: 2 in, 2 out]
            n170 = Add(x=w354, y=w353) -> (x+y=w356:dbl)
            n171 = Subtract(x=w352, y=w354) -> (x-y=w357:dbl)
            n172 = Add(x=w349, y=w354) -> (x+y=w355:dbl)
            n173 = Subtract(x=w351, y=w354) -> (x-y=w350:dbl)
            n174 = Build Array(w352, w353) -> (w359:sgl[])
            n175 = Build Array(w351, w349) -> (w358:sgl[])
            n176 = property on="Stage Position" class="XYGraph (strict)"(error in=w348, "XScale.Maximum"=w356, "XScale.Minimum"=w357, "YScale.Maximum"=w355, "YScale.Minimum"=w350, "XScale.MarkerVals[]"=w359, "YScale.MarkerVals[]"=w358) -> (error out=w334:errorcluster)  [unwired: 1 in, 1 out]
            n177 = local read "EdgePt/nPixelMap"() -> (w338:bool)
            n178 = local read "IDs"() -> (w341:i32[])
            n179 = local read "Step Sizes"() -> (w339:sgl[])
            n180 = local read "Calibration"() -> (w340:cluster{dbl, "MicrostepMode":u32}[])
            n181 = call "SetSyncSettings.vi"("Periodic/nPointScan"=w338, "X SyncOut Enabled"=FALSE, "Y SyncOut Enabled"=FALSE, "error in (no error)"=w334, "Calibration"=w340, "Step Sizes(mm)"=w339, "IDs"=w341) -> ("error out"=w335:errorcluster)  [unwired: 3 in, 1 out]
            n182 = local read "IDs"() -> (w343:i32[])
            n183 = local read "Calibration"() -> (w344:cluster{dbl, "MicrostepMode":u32}[])
            n184 = local write "Next Coordinate Index"(0 ("Next Coordinate Index")) -> ()
            n185 = Build Array(w345, w345) -> (w346:dbl[])
            n186 = Compound Arithmetic op=AND(w329, w328, w327, w326, w325) -> (w324:bool)
            n187 = call "PositionControlRelative.vi"("Mode"=PosCtrlOptions."Both X and Y", "error in (no error)"=w335, "Calibration"=w344, "Move to"=w346, "IDs"=w343) -> ("error out"=w342:errorcluster)  [unwired: 4 in, 2 out]
            n188 = Select(t=StageOptions."Scan_Get Pos", s=w324, f=StageOptions."Idle") -> (s? t:f=w331:T6)
            n189 = local write "Imaging"(w324) -> ()
          }
        }
        n190 = call <vilib>:"Unset Busy.vi"("error in (no error)"=w249) -> ("error out"=w245:errorcluster)  [unwired: 10 in]
      }
      frame "Scan_Get Pos" {
        n191 = local read "IDs"() -> (w373:i32[])
        n192 = local read "Calibration"() -> (w374:cluster{dbl, "MicrostepMode":u32}[])
        n193 = call "PositionControl.vi"("Mode"=PosCtrlOptions."Read Pos", "error in (no error)"=w376, "Calibration"=w374, "IDs"=w373) -> ("error out"=w375:errorcluster, "Moving?"=w365:bool, "Position"=w368:sgl[])  [unwired: 4 in, 1 out]
        n194 = local write "Moving?"(w365) -> ()
        n195 = Index Array(array=w368, index #1=0 ("index"), index #2=1 ("index")) -> (element #1=w362:sgl, element #2=w361:sgl)
        n196 = local write "X Position"(w362) -> ()
        n197 = local write "Y Position"(w361) -> ()
        n198 = Build Array(w362) -> (w371:sgl[])
        n199 = Build Array(w361) -> (w372:sgl[])
        n200 = Bundle(w371, w372) -> (w367:cluster{sgl[], sgl[]})  [unwired: 1 in]
        n201 = local write "Stage Position"(w367) -> ()
        n202 = property on="Stage Position" class="XYGraph (strict)"("Cursor.Cursor X"=w362, "Cursor.Cursor Y"=w361) -> ()  [unwired: 2 in, 2 out]
        n203 = Select(t=StageOptions."Scan_Get Pos", s=w365, f=StageOptions."Scan_SyncSet") -> (s? t:f=w366:T6)
      }
      frame "Scan_SyncSet" {
        n204 = local read "EdgePt/nPixelMap"() -> (w380:bool)
        n205 = local read "IDs"() -> (w388:i32[])
        n206 = local read "Step Sizes"() -> (w386:sgl[])
        n207 = local read "Calibration"() -> (w387:cluster{dbl, "MicrostepMode":u32}[])
        n208 = Quotient & Remainder(x="Next Coordinate Index", y=2) -> (x-y*floor(x/y)=w383:i32)  [unwired: 1 out]
        n209 = Not Equal To 0?(x=w383) -> (x != 0?=w381:bool)
        n210 = Compound Arithmetic op=OR(invert w380, w381) -> (w382:bool)
        n211 = call "SetSyncSettings.vi"("Periodic/nPointScan"=w380, "X SyncOut Enabled"=w382, "Y SyncOut Enabled"=FALSE, "error in (no error)"=w391, "Calibration"=w387, "Step Sizes(mm)"=w386, "IDs"=w388) -> ("error out"=w390:errorcluster)  [unwired: 3 in, 1 out]
      }
      frame "Scan_MoveNext" {
        n212 = flat-sequence {
          tunnel: w405 -> [w408]
          tunnel: [w408] -> w397
          tunnel: [w407] -> w396
          tunnel: [w406] -> w394
          tunnel: [w416] -> w403
          tunnel: [w413] -> w402
          tunnel: [w412] -> w398
          tunnel: w397 -> [w417]
          tunnel: w396 -> [w412]
          tunnel: [w411] -> w395
          tunnel: w394 -> [w411]
          tunnel: [w427] -> w393
          tunnel: [w428] -> w404
          tunnel: w395 -> [w420]
          tunnel: w398 -> [w424]
          tunnel: w402 -> [w425]
          tunnel: w403 -> [w428]
          frame #0 {
            n213 = local read "Machine Mode"() -> (w406:T5)
            n214 = case shown="\"Perimeter Mode\"" w406 {
              tunnel: [w409 w410] -> w407
              frame "Scanning Mode", Default {
                n215 = local read "Coordinate Array"() -> (w409:sgl[][])
              }
              frame "Perimeter Mode" {
                n216 = local read "Peripheral Coordis"() -> (w410:sgl[][])
              }
            }
          }
          frame #1 {
            n217 = local read "IDs"() -> (w415:i32[])
            n218 = local read "Calibration"() -> (w414:cluster{dbl, "MicrostepMode":u32}[])
            n219 = local read "Next Coordinate Index"() -> (w413:i32)
            n220 = Index Array(array=w412, index (row)=w413) -> (element=w418:sgl[])  [unwired: 1 in]
            n221 = call "PositionControl.vi"("Mode"=PosCtrlOptions."Both X and Y", "error in (no error)"=w417, "Calibration"=w414, "Move to"=w418, "IDs"=w415) -> ("error out"=w416:errorcluster)  [unwired: 3 in, 3 out]
          }
          frame #2 {
            n222 = Increment(x=w425) -> (x+1=w421:i32)
            n223 = Matrix Size(0:w424) -> (1:w423:i32)  [unwired: 1 out]
            n224 = Greater?(x=w421, y=w423) -> (0:w422:bool)
            n225 = case shown="True" w422 {
              selector: w422 -> [w429 _]
              tunnel: w421 -> [w430 w433]
              tunnel: [w430 w432] -> w426
              tunnel: [w429 w431] -> w427
              tunnel: w420 -> [_ w434]
              frame False {
              }
              frame True {
                n226 = case shown="\"Perimeter Mode\"" w434 {
                  tunnel: w433 -> [w436 _]
                  tunnel: [w436 0] -> w432
                  tunnel: [TRUE ("x > y?") w438] -> w431
                  frame "Scanning Mode", Default {
                  }
                  frame "Perimeter Mode" {
                    n227 = local read "Outline"() -> (w439:bool)
                    n228 = Not(x=w439) -> (.not. x?=w438:bool)
                  }
                }
              }
            }
            n229 = local write "Next Coordinate Index"(w426) -> ()
          }
        }
        n230 = Not(x=w393) -> (.not. x?=w392:bool)
        n231 = Select(t=StageOptions."Scan_Complete", s=w393, f=StageOptions."Scan_Get Pos") -> (s? t:f=w401:T6)
      }
      frame "Scan_Complete" {
        n232 = stacked-sequence {
          tunnel: [w457 _] -> w444
          tunnel: w442 -> [w449 _]
          frame #0 {
            w446 = FALSE ("Y SyncOut Enabled")
            w455 = 0.0 ("element")
            # "Trigger After Reaching Zero to compensate For a Missed Trigger (If There)"
            n233 = local read "IDs"() -> (w452:i32[])
            n234 = local read "Step Sizes"() -> (w450:sgl[])
            n235 = local read "Calibration"() -> (w451:cluster{dbl, "MicrostepMode":u32}[])
            n236 = call "SetSyncSettings.vi"("Periodic/nPointScan"=w446, "X SyncOut Enabled"=TRUE, "Y SyncOut Enabled"=w446, "error in (no error)"=w449, "Calibration"=w451, "Step Sizes(mm)"=w450, "IDs"=w452) -> ("error out"=w448:errorcluster)  [unwired: 3 in, 1 out]
            n237 = local write "Machine Mode"(T5."Normal" ("Machine Mode")) -> ()
            n238 = local read "IDs"() -> (w453:i32[])
            n239 = local read "Calibration"() -> (w454:cluster{dbl, "MicrostepMode":u32}[])
            n240 = Build Array(w455, w455) -> (w456:dbl[])
            n241 = call "PositionControl.vi"("Mode"=PosCtrlOptions."Both X and Y", "error in (no error)"=w448, "Calibration"=w454, "Move to"=w456, "IDs"=w453) -> ("error out"=w457:errorcluster)  [unwired: 3 in, 3 out]
          }
          frame #1 {
            n242 = local write "Digi Machine Mode"(DigiMachineStates."Idle Mode" ("Digi Machine Mode")) -> ()
          }
        }
      }
      frame "Cmd_MoveAbs" {
        n243 = local read "IDs"() -> (w465:i32[])
        n244 = local read "Calibration"() -> (w464:cluster{dbl, "MicrostepMode":u32}[])
        n245 = Build Array("X Position Abs", "Y Position Abs") -> (w463:dbl[])
        n246 = call "PositionControl.vi"("Mode"=PosCtrlOptions."Both X and Y", "error in (no error)"=w467, "Calibration"=w464, "Move to"=w463, "IDs"=w465) -> ("error out"=w466:errorcluster)  [unwired: 3 in, 3 out]
      }
      frame "Cmd_MoveStart" {
        n247 = local read "X Start"() -> (w470:sgl)
        n248 = local read "Y Start"() -> (w469:sgl)
        n249 = local read "IDs"() -> (w474:i32[])
        n250 = local read "Calibration"() -> (w473:cluster{dbl, "MicrostepMode":u32}[])
        n251 = Build Array(w470, w469) -> (w472:sgl[])
        n252 = call "PositionControl.vi"("Mode"=PosCtrlOptions."Both X and Y", "error in (no error)"=w476, "Calibration"=w473, "Move to"=w472, "IDs"=w474) -> ("error out"=w475:errorcluster)  [unwired: 3 in, 3 out]
      }
      frame "Cmd_CloseControllers" {
        n253 = local read "IDs"() -> (w479:i32[])
        n254 = for {
          shift-right: [w486] -> w483
          shift-left: w481 -> [w485]
          tunnel: w479 -> [w484] mode=indexing
          n255 = call "command stop.vi"("error in (no error)"=w485, "id"=w484) -> ("error out"=w486:errorcluster)  [unwired: 8 in, 1 out]
        }
        n256 = call "CloseDevices.vi"("error in (no error)"=w483, "Close"=TRUE, "Ids"=w479) -> ("error out"=w482:errorcluster)  [unwired: 8 in]
      }
      frame "Cmd_MoveUp" {
        n257 = local read "Move Step"() -> (w490:dbl)
        n258 = local read "IDs"() -> (w489:i32[])
        n259 = local read "Calibration"() -> (w488:cluster{dbl, "MicrostepMode":u32}[])
        n260 = Build Array(0.0 ("element"), w490) -> (w492:dbl[])
        n261 = call "PositionControlRelative.vi"("Mode"=PosCtrlOptions."Move Y", "error in (no error)"=w494, "Calibration"=w488, "Move to"=w492, "IDs"=w489) -> ("error out"=w493:errorcluster)  [unwired: 4 in, 2 out]
      }
      frame "Cmd_MoveDown" {
        n262 = local read "Move Step"() -> (w500:dbl)
        n263 = local read "IDs"() -> (w498:i32[])
        n264 = local read "Calibration"() -> (w497:cluster{dbl, "MicrostepMode":u32}[])
        n265 = Negate(x=w500) -> (-x=w499:dbl)
        n266 = Build Array(0.0 ("element"), w499) -> (w502:dbl[])
        n267 = call "PositionControlRelative.vi"("Mode"=PosCtrlOptions."Move Y", "error in (no error)"=w504, "Calibration"=w497, "Move to"=w502, "IDs"=w498) -> ("error out"=w503:errorcluster)  [unwired: 4 in, 2 out]
      }
      frame "Cmd_MoveLeft" {
        n268 = local read "Move Step"() -> (w511:dbl)
        n269 = local read "IDs"() -> (w507:i32[])
        n270 = local read "Calibration"() -> (w508:cluster{dbl, "MicrostepMode":u32}[])
        n271 = Negate(x=w511) -> (-x=w510:dbl)
        n272 = Build Array(w510, 0.0 ("element")) -> (w512:dbl[])
        n273 = call "PositionControlRelative.vi"("Mode"=PosCtrlOptions."Move X", "error in (no error)"=w514, "Calibration"=w508, "Move to"=w512, "IDs"=w507) -> ("error out"=w513:errorcluster)  [unwired: 4 in, 2 out]
      }
      frame "Cmd_MoveRight" {
        n274 = local read "Move Step"() -> (w520:dbl)
        n275 = local read "IDs"() -> (w518:i32[])
        n276 = local read "Calibration"() -> (w517:cluster{dbl, "MicrostepMode":u32}[])
        n277 = Build Array(w520, 0.0 ("element")) -> (w521:dbl[])
        n278 = call "PositionControlRelative.vi"("Mode"=PosCtrlOptions."Move X", "error in (no error)"=w523, "Calibration"=w517, "Move to"=w521, "IDs"=w518) -> ("error out"=w522:errorcluster)  [unwired: 4 in, 2 out]
      }
      frame "Cmd_MoveZero" {
        w528 = 0.0 ("element")
        n279 = local read "IDs"() -> (w526:i32[])
        n280 = local read "Calibration"() -> (w527:cluster{dbl, "MicrostepMode":u32}[])
        n281 = Build Array(w528, w528) -> (w529:dbl[])
        n282 = call "PositionControl.vi"("Mode"=PosCtrlOptions."Both X and Y", "error in (no error)"=w531, "Calibration"=w527, "Move to"=w529, "IDs"=w526) -> ("error out"=w530:errorcluster)  [unwired: 3 in, 3 out]
      }
      frame "Cmd_GetPos" {
        n283 = local read "IDs"() -> (w543:i32[])
        n284 = local read "Calibration"() -> (w544:cluster{dbl, "MicrostepMode":u32}[])
        n285 = call "PositionControl.vi"("Mode"=PosCtrlOptions."Read Pos", "error in (no error)"=w546, "Calibration"=w544, "IDs"=w543) -> ("error out"=w545:errorcluster, "Moving?"=→"Moving?":bool, "Position"=w537:sgl[])  [unwired: 4 in, 1 out]
        n286 = Index Array(array=w537, index #1=0 ("index"), index #2=1 ("index")) -> (element #1=w534:sgl, element #2=w533:sgl)
        n287 = local write "X Position"(w534) -> ()
        n288 = local write "Y Position"(w533) -> ()
        n289 = Build Array(w534) -> (w541:sgl[])
        n290 = Build Array(w533) -> (w542:sgl[])
        n291 = Bundle(w541, w542) -> (→"Stage Position":cluster{sgl[], sgl[]})  [unwired: 1 in]
        n292 = property on="Stage Position" class="XYGraph (strict)"("Cursor.Cursor X"=w534, "Cursor.Cursor Y"=w533) -> ()  [unwired: 2 in, 2 out]
      }
      frame "Cmd_Stop" {
        n293 = local read "IDs"() -> (w549:i32[])
        n294 = for {
          shift-right: [w554] -> w551
          shift-left: w550 -> [w553]
          tunnel: w549 -> [w552] mode=indexing
          n295 = call "command stop.vi"("error in (no error)"=w553, "id"=w552) -> ("error out"=w554:errorcluster)  [unwired: 8 in, 1 out]
        }
      }
      frame "Sync_On" {
        n296 = local read "EdgePt/nPixelMap"() -> (w557:bool)
        n297 = local read "IDs"() -> (w560:i32[])
        n298 = local read "Step Sizes"() -> (w558:sgl[])
        n299 = local read "Calibration"() -> (w559:cluster{dbl, "MicrostepMode":u32}[])
        n300 = call "SetSyncSettings.vi"("Periodic/nPointScan"=w557, "X SyncOut Enabled"=TRUE, "Y SyncOut Enabled"=FALSE, "error in (no error)"=w563, "Calibration"=w559, "Step Sizes(mm)"=w558, "IDs"=w560) -> ("error out"=w562:errorcluster)  [unwired: 3 in, 1 out]
      }
      frame "Sync_Off" {
        n301 = local read "EdgePt/nPixelMap"() -> (w566:bool)
        n302 = local read "IDs"() -> (w569:i32[])
        n303 = local read "Step Sizes"() -> (w567:sgl[])
        n304 = local read "Calibration"() -> (w568:cluster{dbl, "MicrostepMode":u32}[])
        n305 = call "SetSyncSettings.vi"("Periodic/nPointScan"=w566, "X SyncOut Enabled"=FALSE, "Y SyncOut Enabled"=FALSE, "error in (no error)"=w572, "Calibration"=w568, "Step Sizes(mm)"=w567, "IDs"=w569) -> ("error out"=w571:errorcluster)  [unwired: 3 in, 1 out]
      }
      frame "Stop Motion" {
        w575 = TRUE ("Close")
        n306 = local read "IDs"() -> (w577:i32[])
        n307 = for {
          shift-right: [w583] -> w580
          shift-left: w578 -> [w582]
          tunnel: w577 -> [w581] mode=indexing
          n308 = call "command stop.vi"("error in (no error)"=w582, "id"=w581) -> ("error out"=w583:errorcluster)  [unwired: 8 in, 1 out]
        }
        n309 = call "CloseDevices.vi"("error in (no error)"=w580, "Close"=w575, "Ids"=w577) -> ("error out"=w579:errorcluster)  [unwired: 8 in]
        n310 = local write "Moving?"(FALSE ("Moving?")) -> ()
        n311 = local write "Machine Mode"(T5."Normal" ("Machine Mode")) -> ()
      }
      frame "CloseApplication" {
        w585 = TRUE ("Close")
        n312 = local read "IDs"() -> (w588:i32[])
        n313 = local write "Moving?"(FALSE ("Moving?")) -> ()
        n314 = for {
          shift-right: [w594] -> w591
          shift-left: w589 -> [w593]
          tunnel: w588 -> [w592] mode=indexing
          n315 = call "command stop.vi"("error in (no error)"=w593, "id"=w592) -> ("error out"=w594:errorcluster)  [unwired: 8 in, 1 out]
        }
        n316 = call "CloseDevices.vi"("error in (no error)"=w591, "Close"=w585, "Ids"=w588) -> ("error out"=w590:errorcluster)  [unwired: 8 in]
        n317 = local write "Machine Mode"(T5."Normal" ("Machine Mode")) -> ()
      }
    }
    "Scan Running" <- w56
    n318 = local read "Serial nos"() -> (w62:u32[])
    n319 = call <instrlib>:"Synchronous Latch.vi"("clear"=w70, "set"=w72) -> ("out"=w71:bool)  [unwired: 9 in]
    n320 = call <instrlib>:"Synchronous Latch.vi"("clear"=w57, "set"=w59) -> ("out"=→"Scan Complete":bool)  [unwired: 9 in]
    n321 = Not(x=w71) -> (.not. x?=w64:bool)
    n322 = Greater Than 0?(x=w62) -> (x > 0?=w61:bool[])
    n323 = Or(x=w76, y="Stop Stage") -> (x .or. y?=w73:bool)
    n324 = And Array Elements(Boolean array=w61) -> (logical AND=w60:bool)
    n325 = Select(t=StageOptions."Stop Motion", s=w73, f=w74) -> (s? t:f=w67:T6)
    n326 = And(x=w60, y=w64) -> (x .and. y?=→"Controller Open?":bool)
    n327 = Select(t=StageOptions."CloseApplication", s="Stop Stage App", f=w67) -> (s? t:f=w68:T6)
    "Stage Status" <- w79
  }
  "Error Out Stage" <- w11
  n328 = timed-loop "Generator Control" {
    shift-right: [w603] -> _
    shift-left: Generator_States."Idle" -> [w606]
    shift-right: [w604] -> w25
    shift-left: errorcluster {"status"=FALSE, "code"=0, "source"=""} ("error in") -> [w605]
    timing: w45 -> [_]
    timing-out: [_] -> w44
    stop <- w595 stop-if-true
    n329 = node-c288() -> ()  [unwired: 1 in, 1 out]
    n330 = case shown="\"CloseApp\"" w606 {
      tunnel: [w609 Generator_States."InitGen" Generator_States."Idle" Generator_States."Idle" Generator_States."Idle" Generator_States."Idle"] -> w602
      tunnel: w605 -> [w617 w630 w643 w649 w654 w659]
      tunnel: [w617 w624 w634 w648 w653 w658] -> w604
      tunnel: [_ _ TRUE ("Ext/nViTrig") _ _ _] -> w600
      tunnel: [w616 _ _ _ TRUE ("x .or. y?") w655] -> w599
      tunnel: [_ _ _ _ _ w655] -> w595
      frame "Idle", Default {
        n331 = Build Array("Send vi Trig", "Start Gen", "stop Gen", FALSE ("element")) -> (w615:bool[])
        n332 = Boolean Array To Number(Boolean array=w615) -> (number=w610:u32)
        n333 = case shown="4" w610 {
          tunnel: [Generator_States."Idle" ("f") Generator_States."SendVITrig" Generator_States."GenerateWaveArray" Generator_States."CloseGen"] -> w609
          frame 0, Default {
          }
          frame 1 {
          }
          frame 2 {
          }
          frame 4 {
          }
        }
        n334 = First Call?() -> (First Call?: T/F=w616:bool)
      }
      frame "GenerateWaveArray" {
        n335 = call "WaveSynthV2.vi"("error in"=w630, "Default Wave"="Use Default Wave Settings") -> ("error out"=w624:errorcluster, "Waves per Pixel"=→"Waves per Pixel":u32, "Sampling Frequency (Hz)"=→"Sampling Frequency (Hz)":u64, "Amplitudes"=→"Amplitudes" →"Input Waveform":dbl[], "Offset Factor"=→"Offset Factor":dbl, "Gain"=→"Gain":dbl)  [unwired: 2 in]
      }
      frame "InitGen" {
        n336 = local read "Gain"() -> (w638:dbl)
        n337 = local read "Amplitudes"() -> (w639:dbl[])
        n338 = local read "Sampling Frequency (Hz)"() -> (w641:u64)
        n339 = local read "Waves per Pixel"() -> (w640:u32)
        n340 = local read "Offset Factor"() -> (w637:dbl)
        n341 = call "InitGen.vi"("Offset"=w637, "Gain"=w638, "Ext/nViTrig"="Ext/nViTrig", "Waveform Data Array"=w639, "error in (no error)"=w643, "Wave Per Pixel"=w640, "Sample Rate (Samp/s)"=w641, "FGEN Resource Name"="Generator  Port") -> ("error out"=w635:errorcluster, "Actual Sample Rate"=→"Actual Sample Rate":dbl, "reference out"=w633:refnum<k15>)  [unwired: 1 in]
        n342 = call "EnableOutput.vi"("error in (no error)"=w635, "FGEN Resource Name"=w633) -> ("error out"=w634:errorcluster)  [unwired: 8 in, 1 out]
      }
      frame "SendVITrig" {
        n343 = local read "Generator  Port"() -> (w646:refnum<k15>)
        n344 = call "SendTrig.vi"("error in (no error)"=w649, "Send vi Trig"=TRUE, "Instrument Handle"=w646) -> ("error out"=w648:errorcluster)  [unwired: 7 in, 1 out]
      }
      frame "CloseGen" {
        n345 = local read "Generator  Port"() -> (w652:refnum<k15>)
        n346 = call "CloseGen.vi"("error in (no error)"=w654, "Instrument Handle"=w652) -> ("error out"=w653:errorcluster)  [unwired: 9 in]
      }
      frame "CloseApp" {
        w655 = TRUE ("x .or. y?")
        n347 = local read "Generator  Port"() -> (w657:refnum<k15>)
        n348 = call "CloseGen.vi"("error in (no error)"=w659, "Instrument Handle"=w657) -> ("error out"=w658:errorcluster)  [unwired: 9 in]
      }
    }
    n349 = call <instrlib>:"Synchronous Latch.vi"("clear"=w599, "set"=w600) -> ("out"=→"Generator On":bool)  [unwired: 9 in]
    n350 = Or(x="Stop Gen App", y=w604) -> (x .or. y?=w596:bool)
    n351 = node-c288() -> ()  [unwired: 1 in, 1 out]
    n352 = Select(t=Generator_States."CloseApp", s=w596, f=w602) -> (s? t:f=w603:T4)
    "Gen State" <- w606
  }
  "Error Out Gen" <- w25
  n353 = while {
    stop <- w660 stop-if-true
    n354 = event shown="[1] \"EXIT APP\": Value Change" {
      selector: _ -> [_ _]
      dyn-events: _ -> [_ _]
      timeout: _ -> [_ _]
      tunnel: [_ w664] -> w660
      event Timeout {
        n355 = event-data() -> ()  [unwired: 1 in, 3 out]
      }
      event "EXIT APP": Value Change {
        n356 = event-data() -> ()  [unwired: 1 in, 6 out]
        n357 = flat-sequence {
          tunnel: [w665] -> w663
          tunnel: w663 -> [w668]
          tunnel: [w667] -> w662
          tunnel: w662 -> [w682]
          tunnel: [w681] -> w661
          tunnel: w661 -> [w684]
          tunnel: ["EXIT APP"] -> w664
          frame #0 {
            w666 = TRUE ("Stop Gen App")
            n358 = local write "Stop Stage App"(w666) -> ()
            n359 = local write "Stop Gen App"(w666) -> ()
            n360 = local write "Stop Digi App"(w666) -> ()
            n361 = local write "Stop File App"(w666) -> ()
            n362 = Tick Count (ms)() -> (millisecond timer value=w665:u32)
          }
          frame #1 {
            n363 = while {
              shift-right: [w675] -> _
              shift-left: w668 -> [w675]
              tunnel: [w669] -> w667
              stop <- w672 stop-if-true
              n364 = local read "Generator On"() -> (w680:bool)
              n365 = local read "File Open?"() -> (w679:bool)
              n366 = local read "Digitizer On"() -> (w678:bool)
              n367 = local read "Controller Open?"() -> (w677:bool)
              n368 = Tick Count (ms)() -> (millisecond timer value=w676:u32)
              n369 = Subtract(x=w676, y=w675) -> (x-y=w674:u32)
              n370 = Greater?(x=w674, y=u32 5000) -> (0:w671:bool)
              n371 = Compound Arithmetic op=OR(w680, w679, w678, w677) -> (invert w670:bool)
              n372 = Or(x=w670, y=w671) -> (x .or. y?=w672:bool)
              n373 = Not(x=w670) -> (.not. x?=w669:bool)
            }
          }
          frame #2 {
            w683 = FALSE ("Stop Gen App")
            n374 = call "Display Message to User"("Enable"=w682) -> ("error out"=w681:errorcluster)  [unwired: 9 in, 1 out]
            n375 = local write "Stop Stage App"(w683) -> ()
            n376 = local write "Stop Gen App"(w683) -> ()
            n377 = local write "Stop Digi App"(w683) -> ()
            n378 = local write "Stop File App"(w683) -> ()
          }
          frame #3 {
            w687 = TRUE ("force destroy? (F)")
            n379 = Obtain Queue(name (unnamed)="AquiredDataFIFOCopy", element data type=T9 {"Wave Count"=0, "Wave"=[]} ("input cluster"), create if not found? (T)=TRUE, error in (no error)=w684) -> (queue out=w689:refnum<queue>, error out=w685:errorcluster)  [unwired: 1 in, 1 out]
            n380 = Obtain Queue(name (unnamed)="AquiredDataFIFO", element data type=T9 {"Wave Count"=0, "Wave"=[]} ("input cluster"), create if not found? (T)=TRUE, error in (no error)=w685) -> (queue out=w690:refnum<queue>, error out=w686:errorcluster)  [unwired: 1 in, 1 out]
            n381 = Release Queue(queue=w690, force destroy? (F)=w687, error in (no error)=w686) -> (error out=w688:errorcluster)  [unwired: 2 out]
            n382 = Release Queue(queue=w689, force destroy? (F)=w687, error in (no error)=w688) -> ()  [unwired: 3 out]
          }
          frame #4 {
            n383 = Stop(stop? (T)="EXIT APP") -> ()
          }
        }
      }
    }
  }
  n384 = timed-loop {
    timing: w24 -> [_]
    timing-out: [_] -> w23
    stop <- _ stop-if-true
    n385 = node-c288() -> ()  [unwired: 1 in, 1 out]
    n386 = event shown="[0] Timeout" {
      selector: _ -> [_ _ _ _ _ _]
      dyn-events: _ -> [_ _ _ _ _ _]
      timeout: 0 -> [_ _ _ _ _ _]
      event Timeout {
        w699 = FALSE ("Start Digi")
        n387 = event-data() -> ()  [unwired: 1 in, 3 out]
        n388 = local read "Digi Machine Mode"() -> (w700:T7)
        n389 = local write "Trigger Digi Single"(w699) -> ()
        n390 = local write "Start Digi"(w699) -> ()
        n391 = case shown="\"Scanning Mode\"" w700 {
          frame "Live Mode" {
            w701 = FALSE ("Value (Signaling)")
            n392 = Not(x=w701) -> (.not. x?=w702:bool)
            n393 = local write "Single Shot"(w701) -> ()
            n394 = local write "Scanning"(w701) -> ()
            n395 = local write "LIVE"(w702) -> ()
          }
          frame "Single Shot Mode" {
            w704 = FALSE ("Value (Signaling)")
            n396 = Not(x=w704) -> (.not. x?=w703:bool)
            n397 = local write "Single Shot"(w703) -> ()
            n398 = local write "Scanning"(w704) -> ()
            n399 = local write "LIVE"(w704) -> ()
          }
          frame "Scanning Mode" {
            w706 = FALSE ("Value (Signaling)")
            n400 = Not(x=w706) -> (.not. x?=w705:bool)
            n401 = local write "Single Shot"(w706) -> ()
            n402 = local write "Scanning"(w705) -> ()
            n403 = local write "LIVE"(w706) -> ()
          }
          frame "Idle Mode" {
            w707 = FALSE ("Value (Signaling)")
            n404 = local write "LIVE"(w707) -> ()
            n405 = local write "Single Shot"(w707) -> ()
            n406 = local write "Scanning"(w707) -> ()
          }
        }
      }
      event "TriggerDigi": Value Change {
        n407 = event-data() -> ()  [unwired: 1 in, 6 out]
        n408 = local write "Trigger Digi Single"(TRUE ("Trigger Digi Single")) -> ()
      }
      event "LIVE": Value Change {
        n409 = event-data() -> ()  [unwired: 1 in, 6 out]
        n410 = local write "Digi Machine Mode"(DigiMachineStates."Live Mode" ("Digi Machine Mode")) -> ()
      }
      event "Single Shot": Value Change {
        n411 = event-data() -> ()  [unwired: 1 in, 6 out]
        n412 = local write "Digi Machine Mode"(DigiMachineStates."Single Shot Mode" ("Digi Machine Mode")) -> ()
      }
      event "Scanning": Value Change {
        n413 = event-data() -> ()  [unwired: 1 in, 6 out]
        n414 = local write "Digi Machine Mode"(DigiMachineStates."Scanning Mode" ("Digi Machine Mode")) -> ()
      }
      event "Start Digitizer UI Bttn": Value Change {
        n415 = event-data() -> ()  [unwired: 1 in, 6 out]
        n416 = local write "Start Digi"(TRUE ("Start Digi")) -> ()
      }
    }
    n417 = node-c288() -> ()  [unwired: 1 in, 1 out]
  }
  n418 = node-c288(w23) -> ()  [unwired: 1 out]
  n419 = while {
    stop <- FALSE stop-if-true
    n420 = event shown="[0] \"Save Img\": Value Change" {
      selector: _ -> [_ _]
      dyn-events: _ -> [_ _]
      timeout: 500 -> [_ _]
      event "Save Img": Value Change {
        n421 = event-data() -> ("NewVal"=w717:bool)  [unwired: 1 in, 5 out]
        n422 = case shown="True" w717 {
          frame False {
          }
          frame True {
            w721 = 24
            # "SAVE INTENSITY GRAPH"
            n423 = control-ref of="Image Display"() -> (w718:refnum<vi>)
            n424 = invoke class="IntGraph (strict)" method="Get Image"(reference=w718, "image depth"=w721) -> ("image data"=w735:T20)  [unwired: 4 in, 5 out]
            n425 = local read "FilenameSimeStamped"() -> (w720:string)
            n426 = local read "FileDirectoryFinal"() -> (w719:path)
            n427 = disable-structure shown="Disabled" {
              disable-tunnel: [w745 _] -> w729
              disable-tunnel: w721 -> [w740 _]
              disable-tunnel: w720 -> [w739 _]
              disable-tunnel: w719 -> [w738 _]
              frame Disabled {
                n428 = control-ref of="Topography Plot"() -> (w737:refnum<vi>)
                n429 = invoke class="LabVIEW 3D Graph (strict)" method="Get Image"(reference=w737, "image depth"=w740) -> ("image data"=w746:T20)  [unwired: 4 in, 5 out]
                n430 = Concatenate Strings(w739, "-Index.jpeg" ("string")) -> (w742:string)
                n431 = String To Path(string=w742) -> (path=w741:path)
                n432 = Build Path(base path=w738, name or relative path=w741) -> (appended path=w744:path)
                n433 = call <vilib>:"Write JPEG File.vi"("quality (80)"=100, "image data"=w746, "path to JPEG file"=w744) -> ("error out"=w745:errorcluster)  [unwired: 7 in, 1 out]
              }
              frame Enabled {
              }
            }
            n434 = Concatenate Strings(w720, "-Amplitudes.jpeg" ("string")) -> (w726:string)
            n435 = String To Path(string=w726) -> (path=w727:path)
            n436 = Build Path(base path=w719, name or relative path=w727) -> (appended path=w728:path)
            n437 = call <vilib>:"Write JPEG File.vi"("quality (80)"=100, "image data"=w735, "path to JPEG file"=w728) -> ("error out"=w733:errorcluster)  [unwired: 7 in, 1 out]
            n438 = Merge Errors(w733, w729) -> (w723:errorcluster)
            n439 = Unbundle By Name(w723) -> ("status"=w724:bool)
            n440 = call <vilib>:"Clear Errors.vi"("error in (no error)"=w723, "specific error code to clear (0: all)"=43) -> ("error out"=w731:errorcluster, "specific error cleared?"=w732:bool)  [unwired: 4 in]
            n441 = Not(x=w724) -> (.not. x?=w722:bool)
            n442 = call "Display Message to User2"("error in (no error)"=w731, "Enable"=w732) -> ("error out"=w730:errorcluster)  [unwired: 8 in, 1 out]
            n443 = call "Display Message to User3"("Enable"=w722) -> ()  [unwired: 9 in, 2 out]
            n444 = call <vilib>:"Clear Errors.vi"("error in (no error)"=w730) -> ()  [unwired: 5 in, 2 out]
          }
        }
      }
      event Timeout {
        n445 = event-data() -> ()  [unwired: 1 in, 3 out]
      }
    }
  }
  n446 = node-c288(w44) -> ()  [unwired: 1 out]
  n447 = Obtain Queue(name (unnamed)="AquiredDataFIFO", element data type=T12 {"Wave Count"=0, "Amplitude"=0, "Index"=0} ("cluster"), create if not found? (T)=TRUE) -> (queue out=w41:refnum<queue>, error out=w40:errorcluster)  [unwired: 2 in, 1 out]
  n448 = Obtain Queue(name (unnamed)="AquiredDataFIFO", element data type=T12 {"Wave Count"=0, "Amplitude"=0, "Index"=0} ("cluster"), create if not found? (T)=TRUE) -> (queue out=w2:refnum<queue>, error out=w1:errorcluster)  [unwired: 2 in, 1 out]
  n449 = Obtain Queue(name (unnamed)="AquiredDataFIFOCopy", element data type=T9 {"Wave Count"=0, "Wave"=[]} ("input cluster"), create if not found? (T)=TRUE, error in (no error)=w1) -> (queue out=w26:refnum<queue>, error out=w27:errorcluster)  [unwired: 1 in, 1 out]
  n450 = Obtain Queue(name (unnamed)="AquiredDataFIFO_Wave", element data type=T9 {"Wave Count"=0, "Wave"=[]} ("input cluster"), create if not found? (T)=TRUE) -> (queue out=w14:refnum<queue>, error out=w15:errorcluster)  [unwired: 2 in, 1 out]
  n451 = while "Image View" {
    shift-right: [w755] -> _
    shift-left: w41 -> [w758]
    shift-right: [w754] -> _
    shift-left: w40 -> [w753]
    tunnel: [w757] -> w7
    stop <- w756 stop-if-true
    n452 = call <extravilib>:"Read.vi"("channel"=w757) -> ("element"=w756:bool)  [unwired: 1 in, 1 out]
    n453 = Dequeue Element(queue=w758, timeout in ms (-1)=150, error in (no error)=w753) -> (queue out=w755:refnum<queue>, element=w750:T12, timed out?=w752:bool, error out=w754:errorcluster)
    n454 = case shown="False" w752 {
      tunnel: w750 -> [w767 _]
      frame False {
        n455 = local read "Total Pixels"() -> (w764:i32)
        n456 = Unbundle By Name(w767) -> ("Index"=w759:i32, "Amplitude"=w766:i32, "Wave Count"=w765:i16)
        n457 = Increment(x=w765) -> (x+1=w763:i16)
        n458 = Less Or Equal?(x=w763, y=w764) -> (x <= y?=w760:bool)
        n459 = Compound Arithmetic op=AND(w760, "Imaging") -> (w762:bool)
        n460 = case shown="True" w762 {
          selector: w762 -> [w768 _]
          tunnel: w765 -> [_ w774]
          tunnel: w766 -> [_ w770]
          tunnel: w760 -> [_ _]
          tunnel: w759 -> [_ w769]
          frame False {
            n461 = local write "Imaging"(w768) -> ()
          }
          frame True {
            n462 = local read "Scan Mode"() -> (w772:enum16{"Raster", "Serpentine"})
            n463 = local read "AmplitudeArray"() -> (w781:dbl[])
            n464 = local read "Pixel Count"() -> (w771:i32)
            n465 = call "ImageIndexMap.vi"("Pixel Count"=w771, "Scan Mode"=w772, "Wave Count in"=w774) -> ("Wave Count out"=w773:u32)  [unwired: 8 in]
            n466 = local read "Line Count"() -> (w777:i32)
            n467 = Replace Array Subset(array=w781, new element=w770, index=w773) -> (w779:dbl[])
            n468 = Reshape Array(w779, w777, w771) -> (w776:dbl[][])
            n469 = local write "AmplitudeArray"(w779) -> ()
            n470 = local read "IndexArray"() -> (w780:dbl[])
            n471 = Replace Array Subset(array=w780, new element=w769, index=w773) -> (w778:dbl[])
            n472 = Reshape Array(w778, w777, w771) -> (w775:dbl[][])
            n473 = disable-structure shown="Enabled" {
              disable-tunnel: w776 -> [w785 w793]
              disable-tunnel: w775 -> [w782 _]
              frame Disabled {
                n474 = control-ref of="Scanned Image"() -> (w786:refnum<vi>)
                n475 = call "DisplayImagePlot.vi"("Data Array"=w785, "Picture For Size Ref"=w786, "Colorbar"="ColorBar", "Axis"="Axis", "Map"="Map") -> ("Picture"=→"Scanned Image":picture)  [unwired: 6 in]
                n476 = call <vilib>:"create_plot_surface.vi"("z matrix"=w782) -> ("plots out"=→"Topography Plot":refnum<class "Base Datatype.lvclass">[])  [unwired: 4 in, 6 out]
                n477 = property on="Topography Plot" class="LabVIEW 3D Graph (strict)"("property_graph_fast_draw"=TRUE ("Graph:Fast Draw")) -> ()  [unwired: 2 in, 2 out]
              }
              frame Enabled {
                n478 = local read "X Step Size (R)"() -> (w792:sgl)
                n479 = local read "Y Step Size (R)"() -> (w791:sgl)
                n480 = property on="Image Display" class="IntGraph (strict)"("XScale.Multiplier"=w792, "YScale.Multiplier"=w791) -> ()  [unwired: 2 in, 2 out]
                "Image Display" <- w793
              }
            }
            n481 = local write "IndexArray"(w778) -> ()
          }
        }
      }
      frame True {
      }
    }
    n482 = call "IntensityColorTables.vi"("Map Selector"="Colormap Selector") -> ("Color Map Array"=w748:u32[])  [unwired: 10 in]
    n483 = property on="Image Display" class="IntGraph (strict)"("Color Table"=w748) -> ()  [unwired: 2 in, 2 out]
  }
  n484 = while {
    shift-right: [w807] -> w32
    shift-left: w34 -> [w820]
    shift-right: [w819] -> _
    shift-left: _ -> [w818]
    shift-right: [w809] -> _
    shift-left: Digitizer_StatesMain."Idle" -> [w821]
    shift-right: [w815] -> _
    shift-left: w48 -> [w814]
    shift-right: [w805] -> _
    shift-left: w33 -> [w806]
    shift-right: [w803] -> _
    shift-left: w31 -> [w799]
    tunnel: w7 -> [w796]
    shift-right: [w794] -> _
    shift-left: w19 -> [w795]
    stop <- w797 stop-if-true
    n485 = Equal To 0?(x=w799) -> (x = 0?=→"Wave Count Zero":bool)
    n486 = case shown="\"Read\"" w821 {
      tunnel: w820 -> [w825 w854 w882 w899 w928 w947]
      tunnel: [w825 w834 w875 w898 w914 w945] -> w807
      tunnel: [w829 w846 w865 w893 w918 _] -> w819
      tunnel: w818 -> [w829 _ w867 w894 w921 w946]
      tunnel: [w830 Digitizer_StatesMain."SetParam" ("f") w871 Digitizer_StatesMain."Read" ("f") w923 Digitizer_StatesMain."Idle" ("f")] -> w808
      tunnel: [_ _ w873 _ _ _] -> w816
      tunnel: [w828 _ w869 w895 w922 _] -> w815
      tunnel: w814 -> [w828 _ _ w895 w922 _]
      tunnel: [TRUE _ _ _ _ w944] -> w813
      tunnel: [_ _ _ _ _ w944] -> w798
      tunnel: [w824 w840 w862 w887 w911 w942] -> w805
      tunnel: w806 -> [w824 w839 w862 w887 w912 w942]
      tunnel: [u16 0 ("Wave Count") u16 0 ("Wave Count") w860 w885 w907 u16 0 ("Wave Count")] -> w804
      tunnel: w799 -> [_ _ w861 w885 w904 _]
      tunnel: w795 -> [w822 w837 w857 w884 w903 w940]
      tunnel: [w822 w836 w857 w884 w902 w940] -> w794
      frame "Idle", Default {
        w826 = FALSE ("TIS Configured?")
        n487 = local write "TIS Configured?"(w826) -> ()
        n488 = local write "Configured?"(w826) -> ()
        n489 = Select(t=Digitizer_StatesMain."Init", s="Start Digi", f=Digitizer_StatesMain."Idle") -> (s? t:f=w830:T8)
      }
      frame "Init" {
        n490 = xnode "Open FPGA VI Reference"("error in"=w854, "resource name"="RIO Resource") -> ("FPGA VI Reference Out"=w844:refnum<k20>, "error out"=w853:errorcluster)
        n491 = Type Cast(type=T21 refnum ("FPGA VI Reference Out"), x=w844) -> (*(type *) &x=w843:T21)
        n492 = call "InitDigitizer.vi"("error in"=w853, "FPGA VI Reference In"=w843) -> ("error out"=w848:errorcluster, "range (Vpp)"=→"Range (Vpp)":dbl, "FPGA VI Reference Out"=w849:T21, "TIS Configured?"=→"TIS Configured?":bool, "Configured?"=→"Configured?":bool)  [unwired: 5 in]
        n493 = call "PXITrigReserve-Unreserve.vi"("error in"=w848, "Mode"=enum16{"Reserve", "Unreserve"}."Reserve", "FPGA VI Reference In"=w849) -> ("error out"=w841:errorcluster, "FPGA VI Reference Out"=w846:T21)  [unwired: 7 in]
        n494 = Flush Queue(queue=w839, error in (no error)=w841) -> (queue out=w840:refnum<queue>, error out=w835:errorcluster)  [unwired: 1 out]
        n495 = Flush Queue(queue=w837, error in (no error)=w835) -> (queue out=w836:refnum<queue>, error out=w834:errorcluster)  [unwired: 1 out]
      }
      frame "SetParam" {
        w879 = FALSE  # vi/nGenTrig
        w863 = sgl 5000.0  # ProcessCompletionDelay Factor
        # "Dis-Arm the trigger before seting the parameters! and then Arm Again"
        n496 = local read "Digi Machine Mode"() -> (w868:T7)
        n497 = call "ConfigAquisitionParam.vi"("Requested Samples Per Pixel"="Record Size", "Downsample [0,1,2]"="Time Division", "ProcessCompletionDelay (us)"=w863, "vi/nGenTrig"=w879, "error in"=w882, "AvgCount_powerOf2"="Amplitude \nAveraging", "Delay (us)"="Delay(us)", "FPGA VI Reference In"=w867) -> ("error out"=w877:errorcluster, "Read Size (Host)"=w869:u16, "FPGA VI Reference Out"=w866:T21)  [unwired: 1 in]
        n498 = Equal?(x=w868, y=DigiMachineStates."Scanning Mode") -> (x = y?=w859:bool)
        n499 = Select(t=Digitizer_StatesMain."Read" ("f"), s=w859, f=Digitizer_StatesMain."VITrig") -> (s? t:f=w871:T8)
        n500 = call "Arm(CommitSettings).vi"("Arm?"=TRUE, "error in"=w877, "FPGA VI Reference In"=w866) -> ("error out"=w875:errorcluster, "FPGA VI Reference Out"=w865:T21)  [unwired: 7 in]
        n501 = Unbundle By Name(w875) -> ("status"=w874:bool)
        n502 = Select(t=u16 0, s=w859, f=w861) -> (s? t:f=w860:u16)
        n503 = Not(x=w874) -> (.not. x?=w873:bool)
      }
      frame "VITrig" {
        n504 = Not(x="Pause Triggger") -> (.not. x?=w886:bool)
        n505 = call <instrlib>:"Detect Rising Edge.vi"("signal"="Trigger Digi Single") -> ("edge detected"=w889:bool)  [unwired: 14 in]
        n506 = Equal?(x="Digi Machine Mode", y=DigiMachineStates."Single Shot Mode") -> (x = y?=w891:bool)
        n507 = Select(t=w889, s=w891, f=w886) -> (s? t:f=w888:bool)
        n508 = call "ViTrig.vi"("Vi Trigger"=w888, "error in"=w899, "FPGA VI Reference In"=w894) -> ("error out"=w898:errorcluster, "FPGA VI Reference Out"=w893:T21)  [unwired: 7 in]
        n509 = case shown="True" w886 {
          frame False {
          }
          frame True {
            n510 = Wait (ms)(milliseconds to wait=u32 150) -> ()  [unwired: 1 out]
          }
        }
      }
      frame "Read" {
        n511 = call "ReadFromDigi.vi"("Timeout (ms)"=500, "error in"=w928, "Number of Elements"=w922, "FPGA VI Reference In"=w921) -> ("error out"=w917:errorcluster, "Data Valid?"=w906:bool, "Output Waveform"=w915:u16[], "FPGA VI Reference Out"=w919:T21)  [unwired: 4 in]
        n512 = To Word Integer(number=w915) -> (16bit integer=w910:i16[])
        n513 = Bundle By Name(cluster=T9 {"Wave Count"=0, "Wave"=[]} ("input cluster"), "Wave Count"=w904, "Wave"=w910) -> (w908:T9)
        "Wave out packet" <- w908
        n514 = Increment(x=w904) -> (x+1=w905:u16)
        n515 = call "Arm(CommitSettings).vi"("Arm?"=TRUE, "error in"=w917, "FPGA VI Reference In"=w919) -> ("error out"=w913:errorcluster, "FPGA VI Reference Out"=w918:T21)  [unwired: 7 in]
        n516 = Select(t=w905, s=w906, f=w904) -> (s? t:f=w907:u16)
        n517 = case shown="True" w906 {
          tunnel: w908 -> [_ w933]
          tunnel: w913 -> [w931 w932]
          tunnel: [w931 w934] -> w914
          tunnel: w912 -> [w930 w939]
          tunnel: [w930 w938] -> w911
          tunnel: w903 -> [w929 w937]
          tunnel: [w929 w936] -> w902
          frame False {
          }
          frame True {
            n518 = Enqueue Element(queue=w939, element=w933, error in (no error)=w932) -> (queue out=w938:refnum<queue>, error out=w935:errorcluster)  [unwired: 1 in, 1 out]
            n519 = Enqueue Element(queue=w937, element=w933, error in (no error)=w935) -> (queue out=w936:refnum<queue>, error out=w934:errorcluster)  [unwired: 1 in, 1 out]
          }
        }
        n520 = local read "Digi Machine Mode"() -> (w920:T7)
        n521 = Equal?(x=w920, y=DigiMachineStates."Scanning Mode") -> (x = y?=w926:bool)
        n522 = Select(t=Digitizer_StatesMain."Read" ("f"), s=w926, f=Digitizer_StatesMain."SetParam") -> (s? t:f=w923:T8)
      }
      frame "CloseApp" {
        w944 = TRUE
        n523 = call "PXITrigReserve-Unreserve.vi"("error in"=w947, "Mode"=enum16{"Reserve", "Unreserve"}."Unreserve", "FPGA VI Reference In"=w946) -> ("error out"=w948:errorcluster, "FPGA VI Reference Out"=w949:T21)  [unwired: 7 in]
        n524 = xnode "Close FPGA VI Reference"("FPGA VI Reference In"=w949, "error in"=w948) -> ("error out"=w945:errorcluster)
      }
    }
    n525 = call <vilib>:"Share Stop Signal.vi"("set stop (F)"=w798, "channel"=w796) -> ("stop"=w797:bool)
    "nDigiLoopRunning" <- w797
    n526 = call <instrlib>:"Synchronous Latch.vi"("clear"=w813, "set"=w816) -> ("out"=→"Digitizer On":bool)  [unwired: 9 in]
    n527 = Or(x="Stop Digi App", y=w807) -> (x .or. y?=w811:bool)
    n528 = Select(t=u16 0, s="CountReset", f=w804) -> (s? t:f=w803:u16)
    n529 = Select(t=Digitizer_StatesMain."CloseApp", s=w811, f=w808) -> (s? t:f=w809:T8)
    "Digi State" <- w821
  }
  "error out Digi" <- w32
  n530 = timed-loop "Digitizer UI Handle" {
    timing: w51 -> [_]
    timing-out: [_] -> w50
    tunnel: w7 -> [w952]
    stop <- w951 stop-if-true
    n531 = First Call?() -> (First Call?: T/F=w953:bool)
    n532 = node-c288() -> ()  [unwired: 1 in, 1 out]
    n533 = call <extravilib>:"Read.vi"("channel"=w952) -> ("element"=w951:bool)  [unwired: 1 in, 1 out]
    n534 = case shown="True" w953 {
      frame False {
      }
      frame True {
        n535 = property on="Delay(us)" class="DigNum (strict)"("Val(Sgnl)"=sgl 0.0 ("Value (Signaling)")) -> ()  [unwired: 2 in, 2 out]
      }
    }
    n536 = event shown="[1] \"Amplitude Range\": Value Change" {
      selector: _ -> [_ _ _ _]
      dyn-events: _ -> [_ _ _ _]
      timeout: 0 -> [_ _ _ _]
      event Timeout {
        n537 = event-data() -> ()  [unwired: 1 in, 3 out]
      }
      event "Amplitude Range": Value Change {
        n538 = event-data() -> ("NewVal"=w961:cluster{"Slider 1":dbl, "Slider 1":dbl})  [unwired: 1 in, 5 out]
        n539 = Unbundle(w961) -> ("Slider 1"=w960:dbl, "Slider 1"=w959:dbl)
        n540 = Less?(x=w960, y=w959) -> (x < y?=w958:bool)
        n541 = case shown="True" w958 {
          tunnel: w960 -> [_ w963]
          tunnel: w959 -> [_ w962]
          frame False {
          }
          frame True {
            n542 = property on="Waveform [LIVE]" class="WFGraph (strict)"("YScale.Minimum"=w963, "YScale.Maximum"=w962) -> ()  [unwired: 2 in, 2 out]
          }
        }
      }
      event "FineDelayControl": Value Change {
        n543 = event-data() -> ("OldVal"=w967:dbl, "NewVal"=w968:dbl)  [unwired: 1 in, 4 out]
        n544 = Subtract(x=w968, y=w967) -> (x-y=w966:dbl)
        n545 = property on="Delay(us)" class="DigNum (strict)"() -> ("Value"=w965:sgl)  [unwired: 2 in, 2 out]
        n546 = Add(x=w966, y=w965) -> (x+y=w964:dbl)
        n547 = property on="Delay(us)" class="DigNum (strict)"("Value"=w964) -> ()  [unwired: 2 in, 2 out]
      }
      event "Delay_Scroll_Range", "Delay(us)": Value Change {
        w971 = 0.1 ("Scale.Range:Increment")
        n548 = event-data() -> ()  [unwired: 1 in, 6 out]
        n549 = property on="Delay(us)" class="DigNum (strict)"() -> ("Value"=w969:sgl)  [unwired: 2 in, 2 out]
        n550 = Subtract(x=w969, y="Delay_Scroll_Range") -> (x-y=w973:dbl)
        n551 = Add(x=w969, y="Delay_Scroll_Range") -> (x+y=w972:dbl)
        n552 = property on="FineDelayControl" class="Slide (strict)"("Scale.Increment"=w971, "Scale.MinorInc"=w971, "Scale.Minimum"=w973, "Scale.Maximum"=w972, "Value"=w969) -> ()  [unwired: 2 in, 2 out]
      }
    }
    n553 = node-c288() -> ()  [unwired: 1 in, 1 out]
  }
  n554 = node-c288(w50) -> ()  [unwired: 1 out]
  n555 = while "Wave View" {
    shift-right: [w979] -> _
    shift-left: w14 -> [w982]
    shift-right: [w978] -> _
    shift-left: w15 -> [w977]
    tunnel: w7 -> [w981]
    stop <- w980 stop-if-true
    n556 = call <extravilib>:"Read.vi"("channel"=w981) -> ("element"=w980:bool)  [unwired: 1 in, 1 out]
    n557 = Dequeue Element(queue=w982, timeout in ms (-1)=150, error in (no error)=w977) -> (queue out=w979:refnum<queue>, element=w974:T9, timed out?=w976:bool, error out=w978:errorcluster)
    n558 = case shown="False" w976 {
      tunnel: w974 -> [w997 _]
      frame False {
        n559 = Unbundle By Name(w997) -> ("Wave"=w996:i16[], "Wave Count"=→"Waves Count":u32)
        n560 = local read "Time Division"() -> (w993:u8)
        n561 = control-ref of="Waveform [LIVE]"() -> (w986:refnum<vi>)
        n562 = local read "Range (Vpp)"() -> (w987:dbl)
        n563 = local read "Delay(us)"() -> (w989:sgl)
        n564 = Power Of 2(x=w993) -> (2^x=w992:dbl)
        n565 = Divide(x=1600000000.0 ("Sample Rate"), y=w992) -> (x/y=w991:dbl)
        n566 = call "Scale Acquired Data.vi"("range (V)"=w987, "Start Time (us)"=w989, "Sample Rate"=w991, "Number of Bits"=i16 16, "Data In"=w996) -> ("output waveform"=w988:cluster{"Start Time":dbl, dbl, ext[]})  [unwired: 6 out]
        n567 = call "ShowMinMaxOn Graoh.vi"("Log Mode?"="LogMode", "WaveformGraph in"=w986, "Range (Vpp)"=w987, "output waveform"=w988) -> ("Time (sec)"=→"Max Index (s)":dbl, "Max Abs"=→"Max Val (V)":ext)  [unwired: 4 in, 2 out]
      }
      frame True {
      }
    }
  }
  n568 = while "File I/O Loop" {
    shift-right: [w1002] -> _
    shift-left: Data_Save_State."Idle" -> [w1016]
    shift-right: [w1008] -> w10
    shift-left: w27 -> [w1009]
    shift-right: [w1007] -> _
    shift-left: w38 -> [w1005]
    shift-right: [w1006] -> _
    shift-left: w37 -> [w1004]
    shift-right: [w1000] -> _
    shift-left: w26 -> [w1001]
    shift-right: [w998] -> _
    shift-left: w2 -> [w999]
    stop <- w1003 stop-if-true
    n569 = case shown="\"Open File\"" w1016 {
      tunnel: [w1020 Data_Save_State."Write Attributes" Data_Save_State."Append Data" w1107 Data_Save_State."Idle" Data_Save_State."Idle"] -> w1015
      tunnel: [w1024 _ _ _ TRUE ("Ext/nViTrig") w1125] -> w1011
      tunnel: [_ _ _ _ _ w1125] -> w1003
      tunnel: [_ _ TRUE ("Elements Added?") TRUE ("Elements Added?") _ _] -> w1010
      tunnel: w1009 -> [w1028 w1039 w1073 w1091 w1116 w1129]
      tunnel: [w1028 w1038 w1072 w1077 w1115 w1128] -> w1008
      tunnel: [w1026 w1037 w1071 w1100 w1112 w1124] -> w1007
      tunnel: [w1027 w1036 w1070 w1101 w1111 w1123] -> w1006
      tunnel: w1005 -> [w1026 _ w1074 w1100 w1114 w1127]
      tunnel: w1004 -> [w1027 _ w1070 w1102 w1113 w1126]
      tunnel: w1001 -> [w1025 w1033 w1043 w1095 w1109 w1121]
      tunnel: [w1025 w1033 w1043 w1094 w1109 w1121] -> w1000
      tunnel: w999 -> [w1017 w1030 w1041 w1079 w1108 w1120]
      tunnel: [w1017 w1030 w1041 w1076 w1108 w1120] -> w998
      frame "Idle", Default {
        n570 = Select(t=Data_Save_State."Open File", s="Open File", f=Data_Save_State."Idle") -> (s? t:f=w1029:T10)
        n571 = Select(t=Data_Save_State."Close File", s="Done Recording", f=w1029) -> (s? t:f=w1020:T10)
        n572 = First Call?() -> (First Call?: T/F=w1024:bool)
      }
      frame "Open File" {
        n573 = call "H5_RefOpen.vi"("error in (no error)"=w1039, "Filename"="FileName", "File Directory"="File Store Directory") -> ("error out"=w1038:errorcluster, "HDF5 Dataset Ref out"=w1036:T14, "HDF5 Ref out"=w1037:T14, "FilenameSimeStamped"=→"FilenameSimeStamped":string, "FileDirectoryFinal"=→"FileDirectoryFinal":path)  [unwired: 4 in]
      }
      frame "Write Attributes" {
        n574 = local read "Time Division"() -> (w1060:u8)
        n575 = local read "Sampling Frequency (Hz)"() -> (w1058:u64)
        n576 = local read "Speed Control (mm/s)"() -> (w1064:sgl)
        n577 = local read "Scan Time (Approx.)"() -> (w1051:string)
        n578 = Power Of 2(x=w1060) -> (2^x=w1061:dbl)
        n579 = local read "Waves per Pixel"() -> (w1054:u32)
        n580 = local read "Y Step Size (R)"() -> (w1049:sgl)
        n581 = local read "X Step Size (R)"() -> (w1050:sgl)
        n582 = local read "Amplitudes"() -> (w1056:dbl[])
        n583 = local read "Offset Factor"() -> (w1055:dbl)
        n584 = local read "Pixel Count"() -> (w1063:i32)
        n585 = local read "Record Size"() -> (w1052:u16)
        n586 = local read "Scan Mode"() -> (w1065:enum16{"Raster", "Serpentine"})
        n587 = local read "Line Count"() -> (w1062:i32)
        n588 = local read "Delay(us)"() -> (w1048:sgl)
        n589 = Divide(x=1600000000.0 ("Sample Rate"), y=w1061) -> (x/y=w1053:dbl)
        n590 = local read "X Start"() -> (w1069:sgl)
        n591 = local read "Y Start"() -> (w1067:sgl)
        n592 = local read "X End"() -> (w1068:sgl)
        n593 = local read "Y End"() -> (w1066:sgl)
        n594 = local read "Gain"() -> (w1057:dbl)
        n595 = call "H5_WriteAttr.vi"("HDF5 Ref In"=w1074, "X Start"=w1069, "X End"=w1068, "Y Start"=w1067, "Y End"=w1066, "Scan Mode"=w1065, "Speed Control (mm/s)"=w1064, "error in (no error)"=w1073, "Scan Time (Approx.)"=w1051, "Pixel Count"=w1063, "X Step Size (R)"=w1050, "Line Count"=w1062, "Y Step Size (R)"=w1049, "Gen Sampling Rate"=w1058, "Amplitudes (V)"=w1056, "Offset"=w1055, "Gain"=w1057, "Waves per Pixel"=w1054, "Record Size"=w1052, "Delay(us)"=w1048, "Sampling Freq (Hz)"=w1053, "Temperature"="Temperature (C)", "Remarks"="Remarks", "Transducer Freq(Hz)"="Transducer Freq (Hz)", "Immersion Medium"="Immersion Medium") -> ("HDF5 Ref Out"=w1071:T14, "error out"=w1072:errorcluster)  [unwired: 1 in]
      }
      frame "Append Data" {
        n596 = Dequeue Element(queue=w1095, timeout in ms (-1)=150, error in (no error)=w1091) -> (queue out=w1094:refnum<queue>, element=w1092:T9, timed out?=w1093:bool, error out=w1090:errorcluster)
        n597 = Unbundle By Name(w1092) -> ("Wave"=w1085:i16[], "Wave Count"=w1081:u32)
        n598 = Compound Arithmetic op=AND("Record Data", invert w1093) -> (w1103:bool)
        n599 = Absolute Value(x=w1085) -> (abs(x)=w1086:i16[])
        n600 = call "AppendWaveToFile.vi"("Waveform"=w1085, "error in (no error)"=w1090, "Append?"=w1103, "HDF5 Dataset Ref"=w1102) -> ("error out"=w1078:errorcluster, "HDF5 Dataset out"=w1101:T14)  [unwired: 5 in, 1 out]
        n601 = Array Max & Min(array=w1086) -> (max value=w1082:i16, max index (indices)=w1083:i32)  [unwired: 2 out]
        n602 = local read "Total Pixels"() -> (w1099:i32)
        n603 = Bundle(cluster=T12 {"Wave Count"=0, "Amplitude"=0, "Index"=0}, "Wave Count"=w1081, "Amplitude"=w1082, "Index"=w1083) -> (w1080:T12)
        n604 = local read "Done Recording"() -> (w1088:bool)
        n605 = Increment(x=w1081) -> (x+1=w1087:u32)
        n606 = Greater Or Equal?(x=w1087, y=w1099) -> (x >= y?=w1097:bool)
        "No Trig Miss" <- w1097
        n607 = Or(x=w1088, y=w1097) -> (x .or. y?=w1098:bool)
        n608 = Enqueue Element(queue=w1079, element=w1080, error in (no error)=w1078) -> (queue out=w1076:refnum<queue>, error out=w1077:errorcluster)  [unwired: 1 in, 1 out]
        n609 = Select(t=Data_Save_State."Close File", s=w1098, f=Data_Save_State."Append Data") -> (s? t:f=w1107:T10)
      }
      frame "Close File" {
        w1111 = T14 refnum items=["HDF5 Ref"] ("HDF5 Dataset out")
        w1112 = T14 refnum items=["HDF5 Ref"] ("HDF5 Ref out")
        n610 = call "H5_CloseFile.vi"("error in (no error)"=w1116, "HDF5 Dataset Ref"=w1113, "HDF5 Ref"=w1114) -> ("error out"=w1115:errorcluster)  [unwired: 8 in]
        n611 = flat-sequence {
          frame #0 {
            n612 = property on="Save Img" class="Bool (strict)"("Val(Sgnl)"=TRUE ("Value (Signaling)")) -> ()  [unwired: 2 in, 2 out]
          }
          frame #1 {
            n613 = property on="Save Img" class="Bool (strict)"("Value"=FALSE ("Value (Signaling)")) -> ()  [unwired: 2 in, 2 out]
          }
        }
      }
      frame "Close App" {
        w1123 = T14 refnum items=["HDF5 Ref"] ("HDF5 Dataset out")
        w1124 = T14 refnum items=["HDF5 Ref"] ("HDF5 Ref out")
        w1125 = TRUE ("Ext/nViTrig")
        n614 = call "H5_CloseFile.vi"("error in (no error)"=w1129, "HDF5 Dataset Ref"=w1126, "HDF5 Ref"=w1127) -> ("error out"=w1128:errorcluster)  [unwired: 8 in]
      }
    }
    n615 = call <instrlib>:"Synchronous Latch.vi"("clear"=w1011, "set"=w1010) -> ("out"=→"File Open?":bool)  [unwired: 9 in]
    n616 = Select(t=Data_Save_State."Close App" ("f"), s="Stop File App", f=w1015) -> (s? t:f=w1002:T10)
    "FileStore State" <- w1016
  }
  "Error Out FileIO" <- w10
  n617 = while {
    shift-right: [w1140] -> _
    shift-left: LongShotStates."Idle" -> [w1141]
    shift-right: [w1138] -> _
    shift-left: u8 0 ("Time Division") -> [w1139]
    tunnel: w7 -> [w1136]
    shift-right: [w1135] -> _
    shift-left: _ -> [w1134]
    shift-right: [w1133] -> _
    shift-left: _ -> [w1132]
    shift-right: [w1131] -> _
    shift-left: _ -> [w1130]
    stop <- w1137 stop-if-true
    n618 = call <extravilib>:"Read.vi"() -> ("channel"=w1136:T22, "element"=w1137:bool)  [unwired: 1 in, 1 out]
    n619 = case shown="\"UpdateParam\"" w1141 {
      tunnel: [w1142 w1153 LongShotStates."Take Shot" ("f") w1171 LongShotStates."Set Param" ("f") LongShotStates."Take Shot" ("f") w1202 w1220 LongShotStates."Idle" ("f")] -> w1140
      tunnel: [u8 0 ("Time Division") u8 0 ("Time Division") u8 0 ("Time Division") u8 0 ("Time Division") u8 0 ("Time Division") w1184 w1204 w1216 u8 0 ("Time Division")] -> w1138
      tunnel: w1139 -> [_ _ _ _ _ w1184 w1204 w1217 _]
      tunnel: [_ _ _ _ _ _ w1201 _ _] -> w1135
      tunnel: w1134 -> [_ _ _ _ _ _ w1200 _ _]
      tunnel: [_ _ _ _ _ _ w1197 _ _] -> w1133
      tunnel: w1132 -> [_ _ _ _ _ _ _ w1213 _]
      tunnel: [i16[] [] i16[] [] i16[] [] i16[] [] i16[] [] w1183 w1196 w1212 w1221] -> w1131
      tunnel: w1130 -> [_ _ _ _ _ w1183 w1196 w1211 w1221]
      frame "Idle", Default {
        n620 = Select(t=LongShotStates."Start Gen", s="LongShot", f=LongShotStates."Idle") -> (s? t:f=w1142:T13)
      }
      frame "Start Gen" {
        # "Start Generator"
        n621 = control-ref of="stop Gen"() -> (w1157:refnum<vi>)
        n622 = control-ref of="Generator On"() -> (w1155:refnum<vi>)
        n623 = control-ref of="Start Gen"() -> (w1156:refnum<vi>)
        n624 = call "SwitchTillOn.vi"("Stop if On?"=TRUE, "Turn Off Button"=w1157, "timeout"=u32 300000, "Turn On Button"=w1156, "Turn On Indicator"=w1155) -> ("Success?"=w1152:bool)  [unwired: 6 in]
        n625 = Select(t=LongShotStates."Set Digi Mode", s=w1152, f=LongShotStates."Idle") -> (s? t:f=w1153:T13)
      }
      frame "Set Digi Mode" {
        n626 = flat-sequence {
          frame #0 {
            n627 = local write "Digi Machine Mode"(DigiMachineStates."Single Shot Mode" ("Digi Machine Mode")) -> ()
          }
          frame #1 {
            n628 = while {
              stop <- w1164 stop-if-true
              n629 = local read "Digi Machine Mode"() -> (w1165:T7)
              n630 = Equal?(x=w1165, y=DigiMachineStates."Single Shot Mode") -> (x = y?=w1164:bool)
            }
          }
        }
      }
      frame "Clear Wave Count" {
        # "Reset Wave Number Count"
        n631 = control-ref of="CountReset"() -> (w1175:refnum<vi>)
        n632 = control-ref of="Wave Count Zero"() -> (w1174:refnum<vi>)
        n633 = call "SwitchTillOn.vi"("Stop if On?"=FALSE, "timeout"=u32 5000, "Turn On Button"=w1175, "Turn On Indicator"=w1174) -> ("Success?"=w1170:bool)  [unwired: 7 in]
        n634 = Select(t=LongShotStates."Set Initial Param", s=w1170, f=LongShotStates."Idle") -> (s? t:f=w1171:T13)
      }
      frame "Set Initial Param" {
        w1179 = u16 5 items=["1", "2", "4", "8", "16", "32", "64", "128"] ("Amplitude \nAveraging")
        n635 = local write "Amplitude \nAveraging"(w1179) -> ()
        n636 = local write "Time Division"(u8 2 ("Time Division")) -> ()
        n637 = local write "Record Size"(u16 2048 ("Record Size")) -> ()
        n638 = local write "Delay(us)"(sgl 0.0 ("Delay(us)")) -> ()
      }
      frame "Set Param" {
        n639 = flat-sequence {
          tunnel: w1184 -> [w1188]
          frame #0 {
            n640 = local read "Time Division"() -> (w1190:u8)
            n641 = local read "Record Size"() -> (w1186:u16)
            n642 = Power Of 2(x=w1190) -> (2^x=w1191:dbl)
            n643 = Divide(x=1600000000.0 ("Sample Rate"), y=w1191) -> (x/y=w1187:dbl)
            n644 = Compound Arithmetic op=MULTIPLY(w1186, w1187, w1188) -> (w1192:dbl)
            n645 = local write "Delay(us)"(w1192) -> ()
          }
          frame #1 {
            n646 = while {
              stop <- w1193 stop-if-true
              n647 = local read "Digi State"() -> (w1195:T8)
              n648 = Equal?(x=w1195, y=Digitizer_StatesMain."SetParam") -> (x = y?=w1193:bool)
            }
          }
        }
      }
      frame "Take Shot" {
        n649 = flat-sequence {
          frame #0 {
            n650 = local write "Trigger Digi Single"(FALSE ("Trigger Digi Single")) -> ()
          }
          frame #1 {
            n651 = Wait (ms)(milliseconds to wait=u32 10) -> ()  [unwired: 1 out]
          }
          frame #2 {
            n652 = local write "Trigger Digi Single"(TRUE ("Trigger Digi Single")) -> ()
          }
          frame #3 {
            n653 = Wait (ms)(milliseconds to wait=u32 10) -> ()  [unwired: 1 out]
          }
          frame #4 {
            n654 = local write "Trigger Digi Single"(FALSE ("Trigger Digi Single")) -> ()
          }
        }
        n655 = local read "Wave out packet"() -> (w1203:T9)
        n656 = Unbundle By Name(w1203) -> ("Wave Count"=w1201:u32, "Wave"=w1197:i16[])
        n657 = Greater?(x=w1201, y=w1200) -> (0:w1199:bool)
        n658 = Select(t=LongShotStates."UpdateParam" ("f"), s=w1199, f=LongShotStates."Take Shot") -> (s? t:f=w1202:T13)
      }
      frame "UpdateParam" {
        n659 = Build Array (concatenate)(w1211, w1213) -> (w1212:i16[])
        n660 = Increment(x=w1217) -> (x+1=w1216:u8)
        n661 = Less?(x=w1216, y="LongShotTimes") -> (x < y?=w1214:bool)
        n662 = Select(t=LongShotStates."Set Param", s=w1214, f=LongShotStates."Show Data") -> (s? t:f=w1220:T13)
      }
      frame "Show Data" {
        n663 = call "LongShotView.vi"("Data In"=w1221) -> ()  [unwired: 11 in]
      }
    }
  }
